vi "DOE Gas Volume Consumed.vi"() -> ()   [LabVIEW 2014]
uses:
  <vilib>/DAQmx/read.llb/DAQmx Read (Analog 1D DBL NChan 1Samp).vi
  <vilib>/DAQmx/miscellaneous.llb/DAQmx Fill In Error Info.vi
panel:
  out "25%Sum":dbl
  out "MaxRateSum":dbl
  out "25%RateTime":dbl
  out "MaxRateTime":dbl
  out "CurrentState":string
  in  "Data Sampling Rate (s)":dbl
  out "Second":dbl format="%#.0f"
  out "Minute":dbl format="%#.0f"
  out "25PercentInRange":bool
  out "25PercentRate":bool
  out "MaxRateState":bool
  out "25% Rate Run Average":dbl format="%#.3f"
  out "Target 25% Average":dbl format="%#.3f"
  out "Max Rate Run Avg.":dbl format="%#.3f"
  out "HV":dbl
  out "CF HR":dbl
  out "Meter SLPM":dbl
  out "Sum Time":dbl
  in  "Gas Type":string
  out "Current Meter":dbl
  in  "Reset":bool
  out "Seconds":dbl format="%#.0f"
  out "Minutes":dbl format="%#.0f"
  out "Cubic Ft. Flowed":dbl format="%#.3f"
  out "Signal 2":bool
  out "Reference6":dbl
  out "Reference5":dbl
  out "Reference4":dbl
  out "Reference3":dbl
  out "Reference2":dbl
  out "Reference1":dbl
  in  "HeatingValueLP":dbl=2450.0 min=2400.0 max=2600.0 step=1.0
  out "Output 6":dbl min=0.0 max=5.0 step=0.01
  out "Output 5":dbl min=0.0 max=5.0 step=0.01
  out "Output 4":dbl min=0.0 max=5.0 step=0.01
  out "Output 3":dbl min=0.0 max=5.0 step=0.01
  out "Output 2":dbl min=0.0 max=5.0 step=0.01
  out "Output 1":dbl min=0.0 max=5.0 step=0.01
  in  "HeatingValueNG":dbl=990.0 min=950.0 max=1050.0 step=1.0
  out "Flow Rate":dbl format="%#.0f"
  # "Instant Flow Rate (BTU/hr)"
  # "Heating Value"
  # "Signal"
  # "Elapsed Time"
  # ":"
  # "In Range"
  # "25% Rate Countdown Timer"
  # ":"
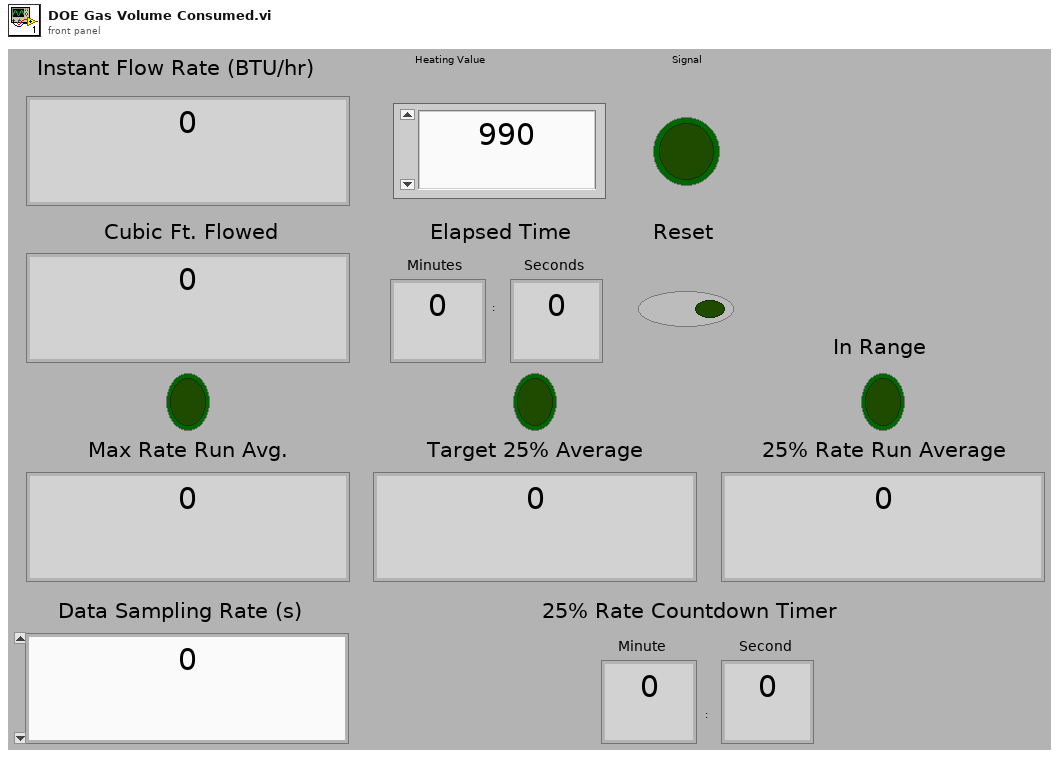
[diagram p1: front panel]
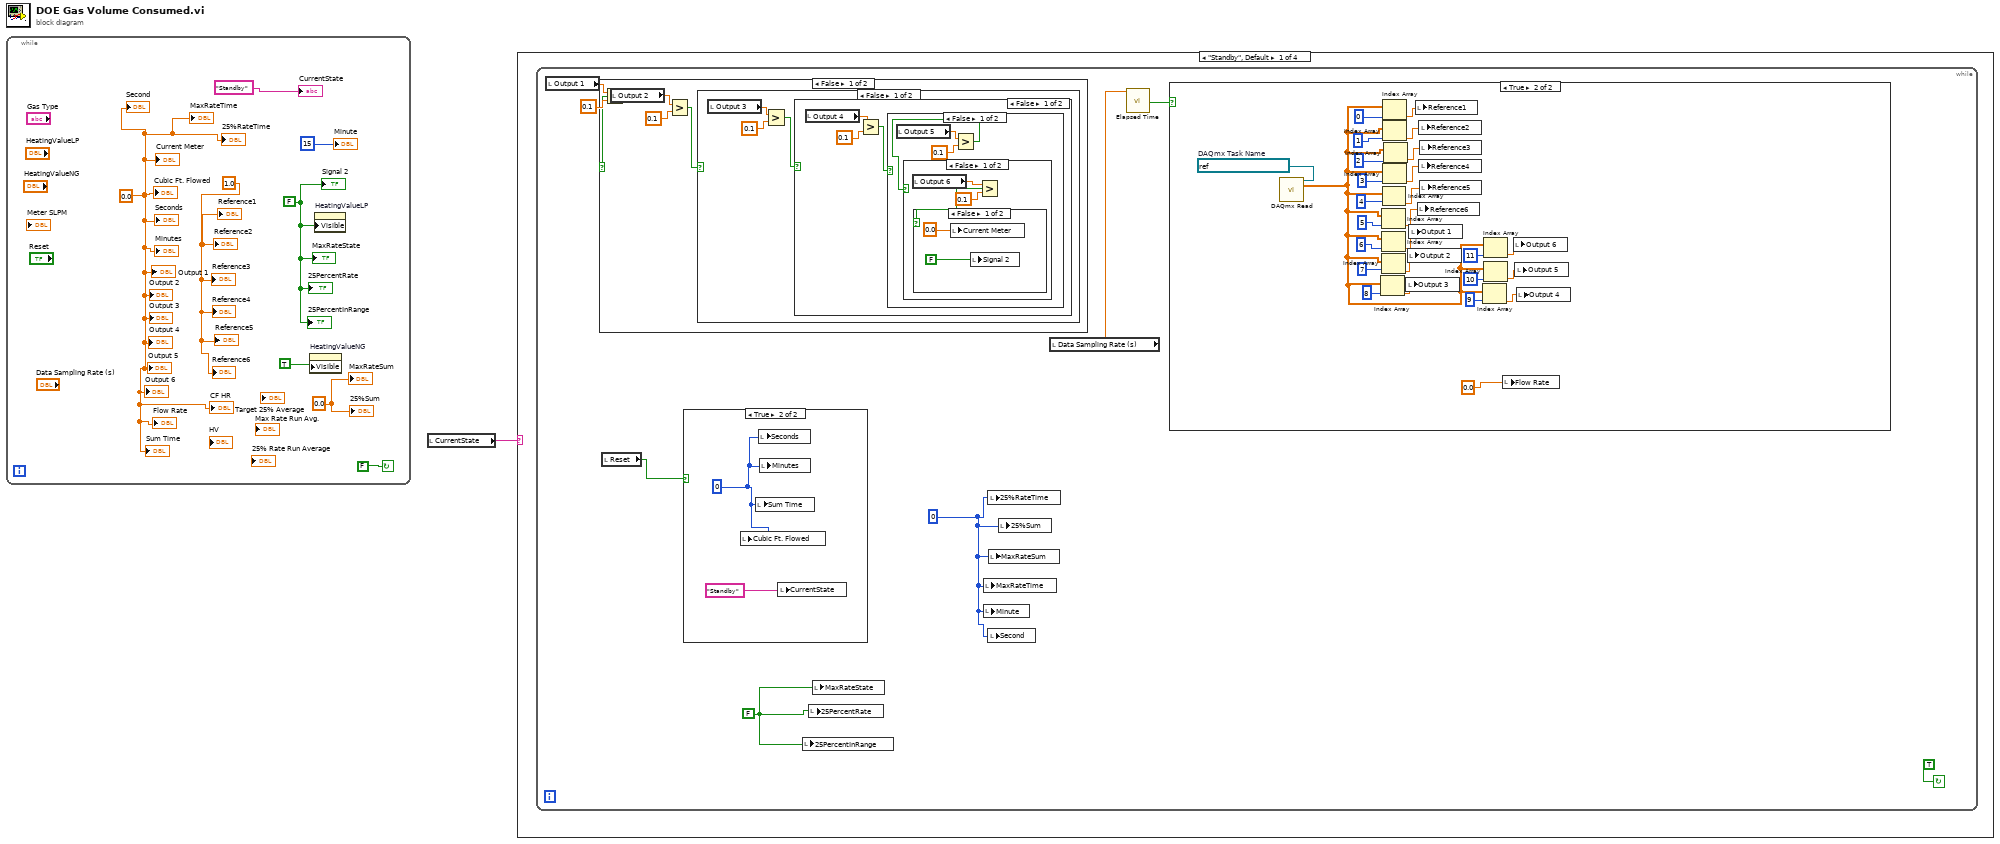
[diagram p0: block diagram]
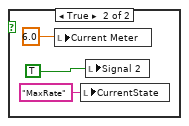
[diagram p3: hidden frame]
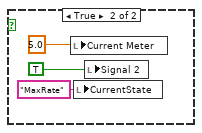
[diagram p4: hidden frame]
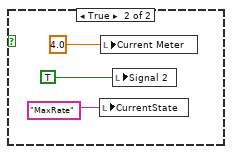
[diagram p5: hidden frame]
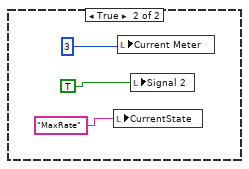
[diagram p6: hidden frame]
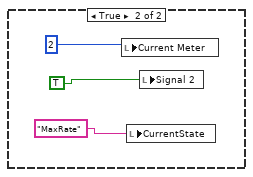
[diagram p7: hidden frame]
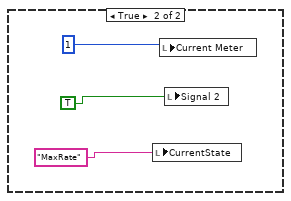
[diagram p8: hidden frame]
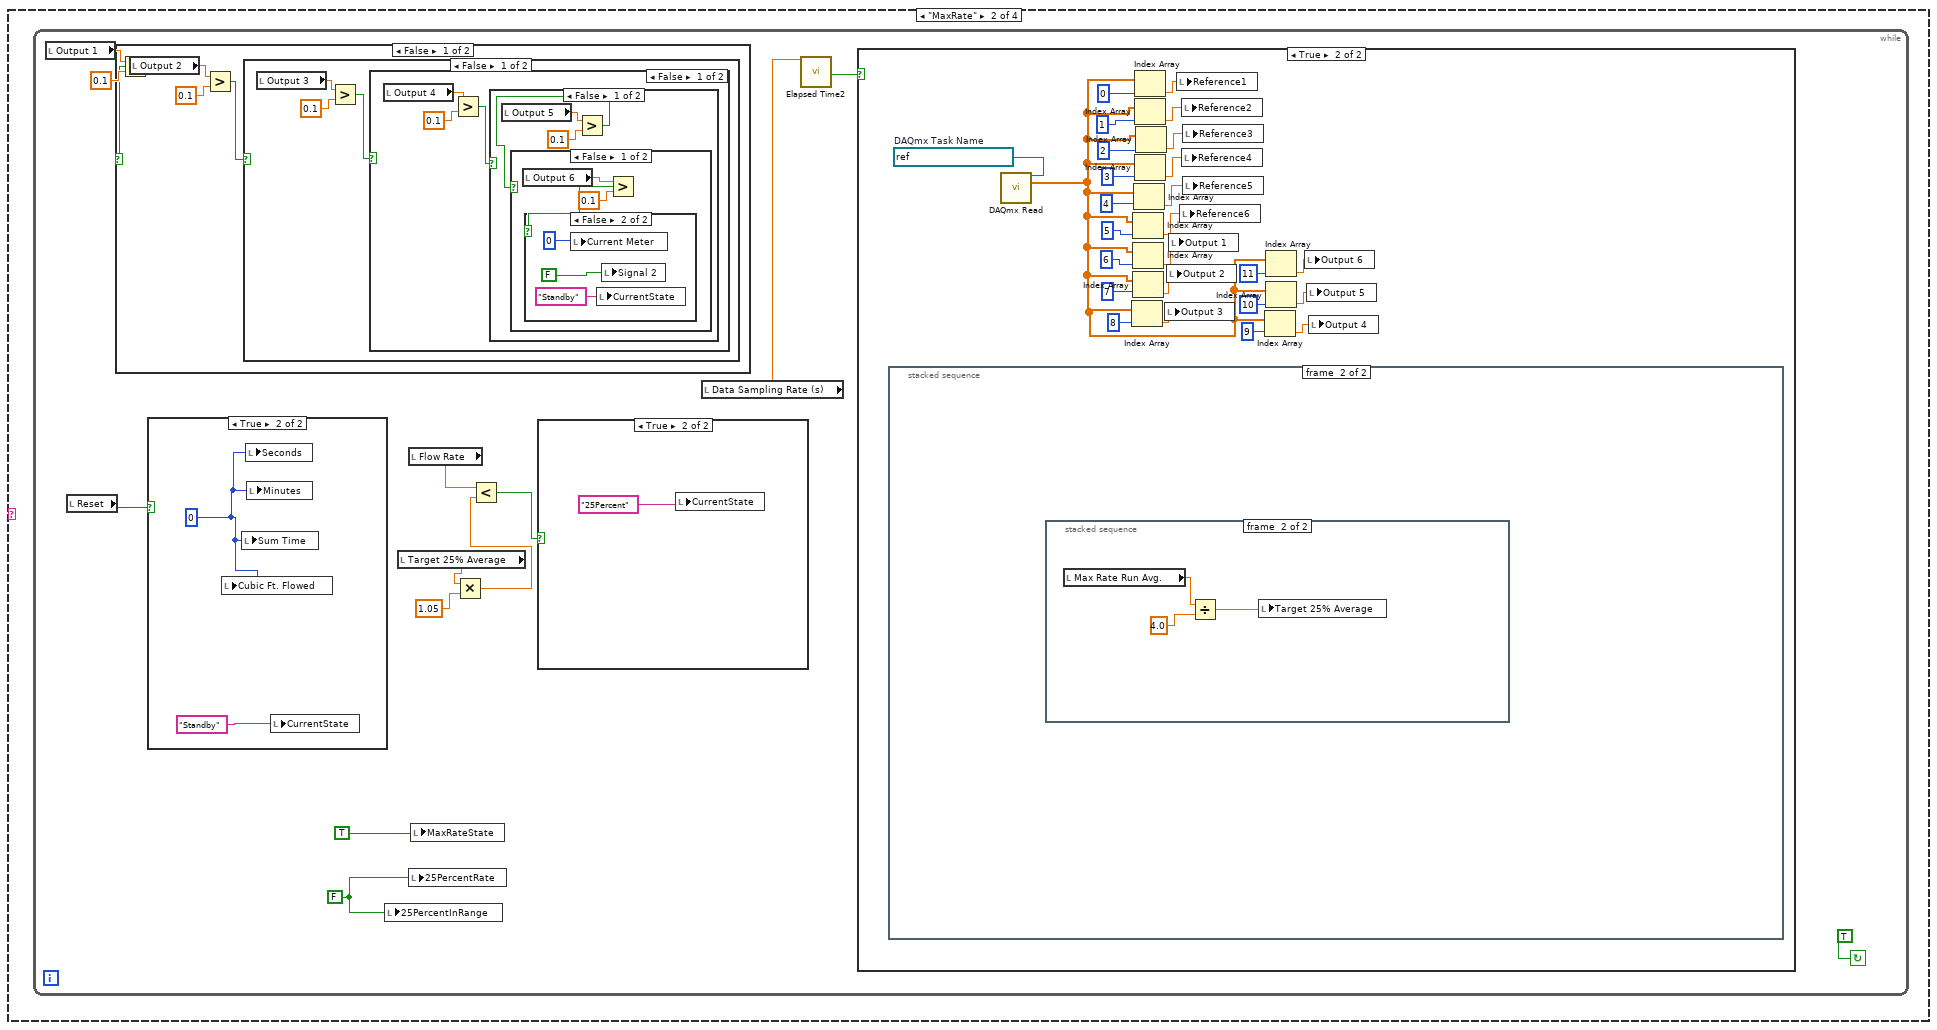
[diagram p10: hidden frame]
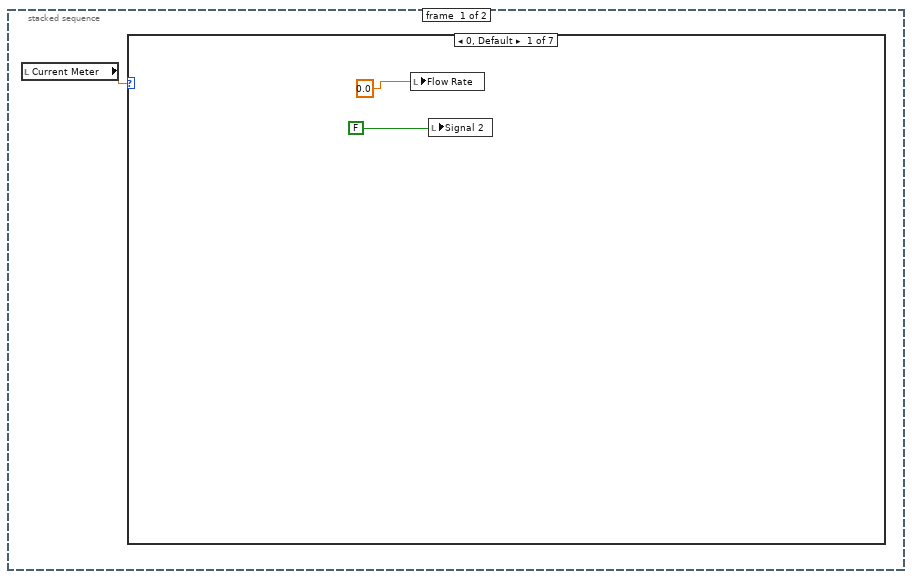
[diagram p13: hidden frame]
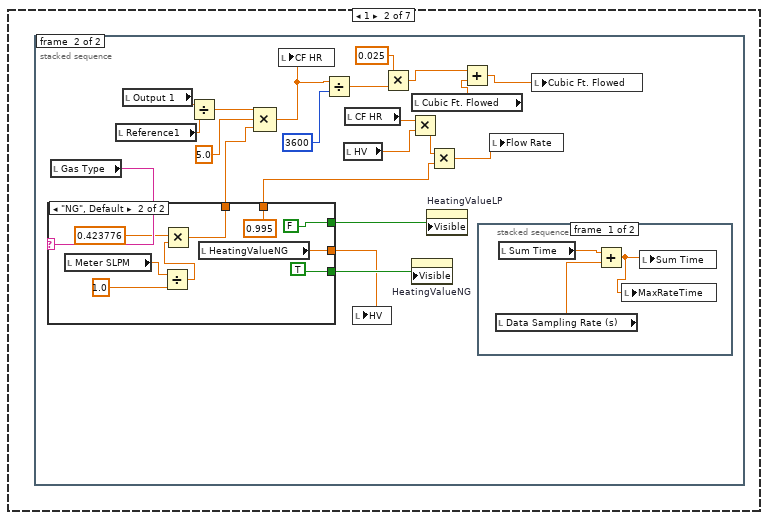
[diagram p14: hidden frame]
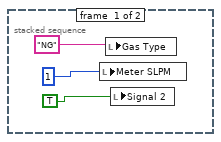
[diagram p15: hidden frame]
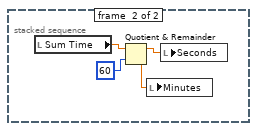
[diagram p16: hidden frame]
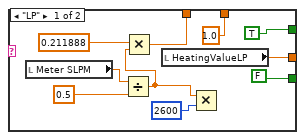
[diagram p17: hidden frame]
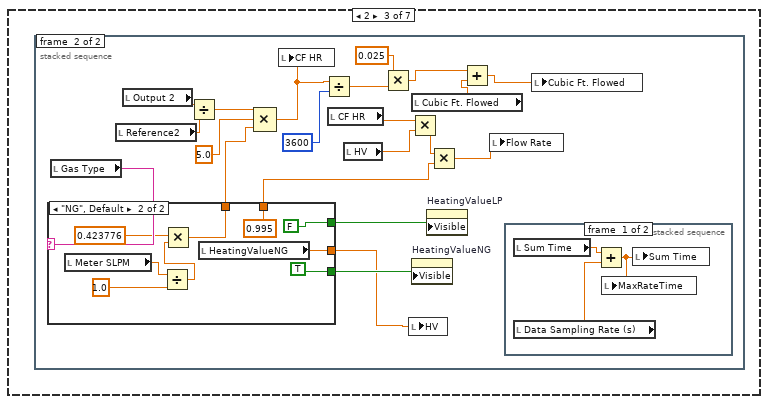
[diagram p18: hidden frame]
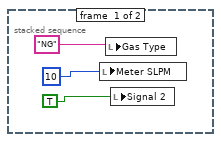
[diagram p19: hidden frame]
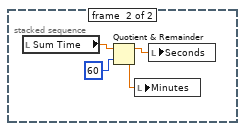
[diagram p20: hidden frame]
diagram:
  n1 = while {
    stop <- FALSE continue-if-true
    w2 = 0.0
    w6 = FALSE
    w9 = 1.0
    w3 = 0.0
    n2 = property on="HeatingValueNG" class="DigNum (strict)"("Visible"=TRUE) -> ()  [unwired: 2 in, 2 out]
    n3 = property on="HeatingValueLP" class="DigNum (strict)"("Visible"=w6) -> ()  [unwired: 2 in, 2 out]
    "Output 1" <- w3
    "Output 2" <- w3
    "Output 3" <- w3
    "Output 4" <- w3
    "Output 5" <- w3
    "Output 6" <- w3
    "Reference1" <- w9
    "Reference2" <- w9
    "Reference3" <- w9
    "Reference4" <- w9
    "Reference5" <- w9
    "Reference6" <- w9
    "Flow Rate" <- w3
    "Signal 2" <- w6
    "Cubic Ft. Flowed" <- w3
    "Minutes" <- w3
    "Seconds" <- w3
    "Current Meter" <- w3
    "Sum Time" <- w3
    "CF HR" <- w3
    "MaxRateState" <- w6
    "25PercentRate" <- w6
    "25PercentInRange" <- w6
    "Minute" <- 15
    "Second" <- w3
    "CurrentState" <- "Standby"
    "25%RateTime" <- w3
    "MaxRateTime" <- w3
    "25%Sum" <- w2
    "MaxRateSum" <- w2
  }
  n4 = local read "CurrentState"() -> (w1:string)
  n5 = case shown="\"Standby\", Default" w1 {
    frame "Standby", Default {
      n6 = while {
        stop <- TRUE continue-if-true
        w10 = 0
        w11 = FALSE
        n7 = local read "Output 1"() -> (w15:dbl)
        n8 = local read "Reset"() -> (w17:bool)
        n9 = Greater?(x=w15, y=0.1) -> (0:w14:bool)
        n10 = case shown="False" w14 {
          frame False {
            n11 = local read "Output 2"() -> (w47:dbl)
            n12 = Greater?(x=w47, y=0.1) -> (0:w46:bool)
            n13 = case shown="False" w46 {
              frame False {
                n14 = local read "Output 3"() -> (w50:dbl)
                n15 = Greater?(x=w50, y=0.1) -> (0:w49:bool)
                n16 = case shown="False" w49 {
                  frame False {
                    n17 = local read "Output 4"() -> (w54:dbl)
                    n18 = Greater?(x=w54, y=0.1) -> (0:w52:bool)
                    n19 = case shown="False" w52 {
                      frame False {
                        n20 = local read "Output 5"() -> (w57:dbl)
                        n21 = Greater?(x=w57, y=0.1) -> (0:w55:bool)
                        n22 = case shown="False" w55 {
                          frame False {
                            n23 = local read "Output 6"() -> (w59:dbl)
                            n24 = Greater?(x=w59, y=0.1) -> (0:w58:bool)
                            n25 = case shown="False" w58 {
                              frame False {
                                n26 = local write "Current Meter"(0.0) -> ()
                                n27 = local write "Signal 2"(FALSE) -> ()
                              }
                              frame True {
                                n28 = local write "Current Meter"(6.0) -> ()
                                n29 = local write "CurrentState"("MaxRate") -> ()
                                n30 = local write "Signal 2"(TRUE) -> ()
                              }
                            }
                          }
                          frame True {
                            n31 = local write "Current Meter"(5.0) -> ()
                            n32 = local write "CurrentState"("MaxRate") -> ()
                            n33 = local write "Signal 2"(TRUE) -> ()
                          }
                        }
                      }
                      frame True {
                        n34 = local write "CurrentState"("MaxRate") -> ()
                        n35 = local write "Current Meter"(4.0) -> ()
                        n36 = local write "Signal 2"(TRUE) -> ()
                      }
                    }
                  }
                  frame True {
                    n37 = local write "CurrentState"("MaxRate") -> ()
                    n38 = local write "Current Meter"(3) -> ()
                    n39 = local write "Signal 2"(TRUE) -> ()
                  }
                }
              }
              frame True {
                n40 = local write "Current Meter"(2) -> ()
                n41 = local write "CurrentState"("MaxRate") -> ()
                n42 = local write "Signal 2"(TRUE) -> ()
              }
            }
          }
          frame True {
            n43 = local write "CurrentState"("MaxRate") -> ()
            n44 = local write "Current Meter"(1) -> ()
            n45 = local write "Signal 2"(TRUE) -> ()
          }
        }
        n46 = case shown="True" w17 {
          frame False {
          }
          frame True {
            w82 = 0
            n47 = local write "Cubic Ft. Flowed"(w82) -> ()
            n48 = local write "Sum Time"(w82) -> ()
            n49 = local write "Seconds"(w82) -> ()
            n50 = local write "Minutes"(w82) -> ()
            n51 = local write "CurrentState"("Standby") -> ()
          }
        }
        n52 = local write "25PercentInRange"(w11) -> ()
        n53 = local write "25PercentRate"(w11) -> ()
        n54 = local write "MaxRateState"(w11) -> ()
        n55 = local write "MaxRateTime"(w10) -> ()
        n56 = local write "Minute"(w10) -> ()
        n57 = local write "25%RateTime"(w10) -> ()
        n58 = local write "Second"(w10) -> ()
        n59 = local write "MaxRateSum"(w10) -> ()
        n60 = local write "25%Sum"(w10) -> ()
        n61 = local read "Data Sampling Rate (s)"() -> (w12:dbl)
        n62 = call "Elapsed Time"("Time Target (s)"=w12) -> ("Time has Elapsed"=w13:bool)  [unwired: 11 in, 7 out]
        n63 = case shown="True" w13 {
          frame False {
          }
          frame True {
            w45 = refnum<k21> "ReadFlowMeterIn"  # DAQmx Task Name
            n64 = call-poly <vilib>:"DAQmx Read.vi"("task/channels in"=w45) -> ("data"=w44:dbl[])  [unwired: 12 in, 2 out]
            n65 = Index Array(array=w44, index=8) -> (element=w28:dbl)
            n66 = Index Array(array=w44, index=5) -> (element=w25:dbl)
            n67 = Index Array(array=w44, index=6) -> (element=w26:dbl)
            n68 = Index Array(array=w44, index=7) -> (element=w27:dbl)
            n69 = Index Array(array=w44, index=4) -> (element=w24:dbl)
            n70 = Index Array(array=w44, index=0) -> (element=w20:dbl)
            n71 = Index Array(array=w44, index=1) -> (element=w21:dbl)
            n72 = Index Array(array=w44, index=3) -> (element=w23:dbl)
            n73 = Index Array(array=w44, index=2) -> (element=w22:dbl)
            n74 = local write "Output 3"(w28) -> ()
            n75 = local write "Output 2"(w27) -> ()
            n76 = local write "Output 1"(w26) -> ()
            n77 = local write "Reference1"(w20) -> ()
            n78 = local write "Reference6"(w25) -> ()
            n79 = local write "Reference2"(w21) -> ()
            n80 = local write "Reference4"(w23) -> ()
            n81 = local write "Reference3"(w22) -> ()
            n82 = local write "Reference5"(w24) -> ()
            n83 = Index Array(array=w44, index=9) -> (element=w29:dbl)
            n84 = Index Array(array=w44, index=11) -> (element=w31:dbl)
            n85 = Index Array(array=w44, index=10) -> (element=w30:dbl)
            n86 = local write "Flow Rate"(0.0) -> ()
            n87 = local write "Output 6"(w31) -> ()
            n88 = local write "Output 5"(w30) -> ()
            n89 = local write "Output 4"(w29) -> ()
          }
        }
      }
    }
    frame "MaxRate" {
      n90 = while {
        stop <- TRUE continue-if-true
        w88 = FALSE
        n91 = local read "Output 1"() -> (w93:dbl)
        n92 = local read "Reset"() -> (w95:bool)
        n93 = Greater?(x=w93, y=0.1) -> (0:w92:bool)
        n94 = case shown="False" w92 {
          frame False {
            n95 = local read "Output 2"() -> (w436:dbl)
            n96 = Greater?(x=w436, y=0.1) -> (0:w435:bool)
            n97 = case shown="False" w435 {
              frame False {
                n98 = local read "Output 3"() -> (w439:dbl)
                n99 = Greater?(x=w439, y=0.1) -> (0:w438:bool)
                n100 = case shown="False" w438 {
                  frame False {
                    n101 = local read "Output 4"() -> (w443:dbl)
                    n102 = Greater?(x=w443, y=0.1) -> (0:w441:bool)
                    n103 = case shown="False" w441 {
                      frame False {
                        n104 = local read "Output 5"() -> (w446:dbl)
                        n105 = Greater?(x=w446, y=0.1) -> (0:w444:bool)
                        n106 = case shown="False" w444 {
                          frame False {
                            n107 = local read "Output 6"() -> (w448:dbl)
                            n108 = Greater?(x=w448, y=0.1) -> (0:w447:bool)
                            n109 = case shown="False" w447 {
                              frame True {
                                n110 = local write "Current Meter"(6.0) -> ()
                                n111 = local write "Signal 2"(TRUE) -> ()
                              }
                              frame False {
                                n112 = local write "Current Meter"(0) -> ()
                                n113 = local write "CurrentState"("Standby") -> ()
                                n114 = local write "Signal 2"(FALSE) -> ()
                              }
                            }
                          }
                          frame True {
                            n115 = local write "Current Meter"(5.0) -> ()
                            n116 = local write "Signal 2"(TRUE) -> ()
                          }
                        }
                      }
                      frame True {
                        n117 = local write "Current Meter"(4.0) -> ()
                        n118 = local write "Signal 2"(TRUE) -> ()
                      }
                    }
                  }
                  frame True {
                    n119 = local write "Current Meter"(3) -> ()
                    n120 = local write "Signal 2"(TRUE) -> ()
                  }
                }
              }
              frame True {
                n121 = local write "Current Meter"(2) -> ()
                n122 = local write "Signal 2"(TRUE) -> ()
              }
            }
          }
          frame True {
            n123 = local write "Current Meter"(1) -> ()
            n124 = local write "Signal 2"(TRUE) -> ()
          }
        }
        n125 = case shown="True" w95 {
          frame False {
          }
          frame True {
            w466 = 0
            n126 = local write "Cubic Ft. Flowed"(w466) -> ()
            n127 = local write "Sum Time"(w466) -> ()
            n128 = local write "Seconds"(w466) -> ()
            n129 = local write "Minutes"(w466) -> ()
            n130 = local write "CurrentState"("Standby") -> ()
          }
        }
        n131 = local write "25PercentInRange"(w88) -> ()
        n132 = local read "Target 25% Average"() -> (w85:dbl)
        n133 = local read "Flow Rate"() -> (w87:dbl)
        n134 = local write "25PercentRate"(w88) -> ()
        n135 = local write "MaxRateState"(TRUE) -> ()
        n136 = Multiply(x=w85, y=1.05) -> (x*y=w84:dbl)
        n137 = Less?(x=w87, y=w84) -> (x < y?=w83:bool)
        n138 = case shown="True" w83 {
          frame False {
          }
          frame True {
            n139 = local write "CurrentState"("25Percent") -> ()
          }
        }
        n140 = local read "Data Sampling Rate (s)"() -> (w90:dbl)
        n141 = call "Elapsed Time2"("Time Target (s)"=w90) -> ("Time has Elapsed"=w91:bool)  [unwired: 11 in, 7 out]
        n142 = case shown="True" w91 {
          frame False {
          }
          frame True {
            w123 = refnum<k21> "ReadFlowMeterIn"  # DAQmx Task Name
            n143 = stacked-sequence {
              frame #0 {
                n144 = local read "Current Meter"() -> (w124:dbl)
                n145 = case shown="0, Default" w124 {
                  frame 0, Default {
                    n146 = local write "Flow Rate"(0.0) -> ()
                    n147 = local write "Signal 2"(FALSE) -> ()
                  }
                  frame 1 {
                    n148 = stacked-sequence {
                      frame #0 {
                        n149 = local write "Meter SLPM"(1) -> ()
                        n150 = local write "Gas Type"("NG") -> ()
                        n151 = local write "Signal 2"(TRUE) -> ()
                      }
                      frame #1 {
                        n152 = local read "Gas Type"() -> (w142:string)
                        n153 = case shown="\"NG\", Default" w142 {
                          tunnel: [w164 w173] -> w141
                          tunnel: [TRUE FALSE] -> w140
                          tunnel: [FALSE TRUE] -> w139
                          tunnel: [1.0 0.995] -> w138
                          tunnel: [w158 w168] -> w137
                          frame "LP" {
                            n154 = local read "Meter SLPM"() -> (w166:dbl)
                            n155 = Divide(x=w166, y=0.5) -> (x/y=w159:dbl)
                            n156 = Multiply(x=0.211888, y=w159) -> (x*y=w164:dbl)
                            n157 = local read "HeatingValueLP"() -> (w158:dbl)
                            n158 = Multiply(x=w159, y=2600) -> ()  [unwired: 1 out]
                          }
                          frame "NG", Default {
                            n159 = local read "Meter SLPM"() -> (w175:dbl)
                            n160 = Divide(x=w175, y=1.0) -> (x/y=w169:dbl)
                            n161 = Multiply(x=0.423776, y=w169) -> (x*y=w173:dbl)
                            n162 = local read "HeatingValueNG"() -> (w168:dbl)
                          }
                        }
                        n163 = local read "Reference1"() -> (w145:dbl)
                        n164 = local read "Output 1"() -> (w146:dbl)
                        n165 = Divide(x=w146, y=w145) -> (x/y=w143:dbl)
                        n166 = Compound Arithmetic op=MULTIPLY(w143, 5.0, w141) -> (w136:dbl)
                        n167 = local write "CF HR"(w136) -> ()
                        n168 = Divide(x=w136, y=3600) -> (x/y=w134:dbl)
                        n169 = local read "HV"() -> (w148:dbl)
                        n170 = local read "CF HR"() -> (w147:dbl)
                        n171 = local write "HV"(w137) -> ()
                        n172 = Multiply(x=0.025, y=w134) -> (x*y=w131:dbl)
                        n173 = Multiply(x=w147, y=w148) -> (x*y=w149:dbl)
                        n174 = local read "Cubic Ft. Flowed"() -> (w132:dbl)
                        n175 = property on="HeatingValueNG" class="DigNum (strict)"("Visible"=w139) -> ()  [unwired: 2 in, 2 out]
                        n176 = property on="HeatingValueLP" class="DigNum (strict)"("Visible"=w140) -> ()  [unwired: 2 in, 2 out]
                        n177 = Multiply(x=w149, y=w138) -> (x*y=w150:dbl)
                        n178 = Add(x=w131, y=w132) -> (x+y=w130:dbl)
                        n179 = stacked-sequence {
                          frame #0 {
                            n180 = local read "Data Sampling Rate (s)"() -> (w152:dbl)
                            n181 = local read "Sum Time"() -> (w153:dbl)
                            n182 = Add(x=w153, y=w152) -> (x+y=w151:dbl)
                            n183 = local write "MaxRateTime"(w151) -> ()
                            n184 = local write "Sum Time"(w151) -> ()
                          }
                          frame #1 {
                            n185 = local read "Sum Time"() -> (w157:dbl)
                            n186 = Quotient & Remainder(x=w157, y=60) -> (x-y*floor(x/y)=w154:dbl, floor(x/y)=w155:dbl)
                            n187 = local write "Minutes"(w155) -> ()
                            n188 = local write "Seconds"(w154) -> ()
                          }
                        }
                        n189 = local write "Flow Rate"(w150) -> ()
                        n190 = local write "Cubic Ft. Flowed"(w130) -> ()
                      }
                    }
                  }
                  frame 2 {
                    n191 = stacked-sequence {
                      frame #0 {
                        n192 = local write "Meter SLPM"(10) -> ()
                        n193 = local write "Gas Type"("NG") -> ()
                        n194 = local write "Signal 2"(TRUE) -> ()
                      }
                      frame #1 {
                        n195 = local read "Gas Type"() -> (w192:string)
                        n196 = case shown="\"NG\", Default" w192 {
                          tunnel: [w214 w223] -> w191
                          tunnel: [TRUE FALSE] -> w190
                          tunnel: [FALSE TRUE] -> w189
                          tunnel: [1.0 0.995] -> w188
                          tunnel: [w208 w218] -> w187
                          frame "LP" {
                            n197 = local read "Meter SLPM"() -> (w216:dbl)
                            n198 = Divide(x=w216, y=0.5) -> (x/y=w209:dbl)
                            n199 = Multiply(x=0.211888, y=w209) -> (x*y=w214:dbl)
                            n200 = local read "HeatingValueLP"() -> (w208:dbl)
                            n201 = Multiply(x=w209, y=2600) -> ()  [unwired: 1 out]
                          }
                          frame "NG", Default {
                            n202 = local read "Meter SLPM"() -> (w225:dbl)
                            n203 = Divide(x=w225, y=1.0) -> (x/y=w219:dbl)
                            n204 = Multiply(x=0.423776, y=w219) -> (x*y=w223:dbl)
                            n205 = local read "HeatingValueNG"() -> (w218:dbl)
                          }
                        }
                        n206 = local read "Reference2"() -> (w195:dbl)
                        n207 = local read "Output 2"() -> (w196:dbl)
                        n208 = Divide(x=w196, y=w195) -> (x/y=w193:dbl)
                        n209 = Compound Arithmetic op=MULTIPLY(w193, 5.0, w191) -> (w186:dbl)
                        n210 = local write "CF HR"(w186) -> ()
                        n211 = Divide(x=w186, y=3600) -> (x/y=w184:dbl)
                        n212 = local read "CF HR"() -> (w197:dbl)
                        n213 = local read "HV"() -> (w198:dbl)
                        n214 = Multiply(x=0.025, y=w184) -> (x*y=w181:dbl)
                        n215 = local write "HV"(w187) -> ()
                        n216 = Multiply(x=w197, y=w198) -> (x*y=w199:dbl)
                        n217 = local read "Cubic Ft. Flowed"() -> (w182:dbl)
                        n218 = property on="HeatingValueNG" class="DigNum (strict)"("Visible"=w189) -> ()  [unwired: 2 in, 2 out]
                        n219 = property on="HeatingValueLP" class="DigNum (strict)"("Visible"=w190) -> ()  [unwired: 2 in, 2 out]
                        n220 = Multiply(x=w199, y=w188) -> (x*y=w200:dbl)
                        n221 = Add(x=w181, y=w182) -> (x+y=w180:dbl)
                        n222 = local write "Flow Rate"(w200) -> ()
                        n223 = stacked-sequence {
                          frame #0 {
                            n224 = local read "Sum Time"() -> (w203:dbl)
                            n225 = local read "Data Sampling Rate (s)"() -> (w202:dbl)
                            n226 = Add(x=w203, y=w202) -> (x+y=w201:dbl)
                            n227 = local write "MaxRateTime"(w201) -> ()
                            n228 = local write "Sum Time"(w201) -> ()
                          }
                          frame #1 {
                            n229 = local read "Sum Time"() -> (w207:dbl)
                            n230 = Quotient & Remainder(x=w207, y=60) -> (x-y*floor(x/y)=w204:dbl, floor(x/y)=w205:dbl)
                            n231 = local write "Minutes"(w205) -> ()
                            n232 = local write "Seconds"(w204) -> ()
                          }
                        }
                        n233 = local write "Cubic Ft. Flowed"(w180) -> ()
                      }
                    }
                  }
                  frame 3 {
                    n234 = stacked-sequence {
                      frame #0 {
                        n235 = local write "Meter SLPM"(20) -> ()
                        n236 = local write "Gas Type"("NG") -> ()
                        n237 = local write "Signal 2"(TRUE) -> ()
                      }
                      frame #1 {
                        n238 = local read "Gas Type"() -> (w242:string)
                        n239 = case shown="\"NG\", Default" w242 {
                          tunnel: [w264 w273] -> w241
                          tunnel: [TRUE FALSE] -> w240
                          tunnel: [FALSE TRUE] -> w239
                          tunnel: [1.0 0.995] -> w238
                          tunnel: [w258 w268] -> w237
                          frame "LP" {
                            n240 = local read "Meter SLPM"() -> (w266:dbl)
                            n241 = Divide(x=w266, y=0.5) -> (x/y=w259:dbl)
                            n242 = Multiply(x=0.211888, y=w259) -> (x*y=w264:dbl)
                            n243 = local read "HeatingValueLP"() -> (w258:dbl)
                            n244 = Multiply(x=w259, y=2600) -> ()  [unwired: 1 out]
                          }
                          frame "NG", Default {
                            n245 = local read "Meter SLPM"() -> (w275:dbl)
                            n246 = Divide(x=w275, y=1.0) -> (x/y=w269:dbl)
                            n247 = Multiply(x=0.423776, y=w269) -> (x*y=w273:dbl)
                            n248 = local read "HeatingValueNG"() -> (w268:dbl)
                          }
                        }
                        n249 = local read "Reference3"() -> (w245:dbl)
                        n250 = local read "Output 3"() -> (w246:dbl)
                        n251 = Divide(x=w246, y=w245) -> (x/y=w243:dbl)
                        n252 = Compound Arithmetic op=MULTIPLY(w243, 5.0, w241) -> (w236:dbl)
                        n253 = local write "CF HR"(w236) -> ()
                        n254 = Divide(x=w236, y=3600) -> (x/y=w234:dbl)
                        n255 = local read "CF HR"() -> (w247:dbl)
                        n256 = local read "HV"() -> (w248:dbl)
                        n257 = Multiply(x=0.025, y=w234) -> (x*y=w231:dbl)
                        n258 = local write "HV"(w237) -> ()
                        n259 = Multiply(x=w247, y=w248) -> (x*y=w249:dbl)
                        n260 = local read "Cubic Ft. Flowed"() -> (w232:dbl)
                        n261 = property on="HeatingValueNG" class="DigNum (strict)"("Visible"=w239) -> ()  [unwired: 2 in, 2 out]
                        n262 = property on="HeatingValueLP" class="DigNum (strict)"("Visible"=w240) -> ()  [unwired: 2 in, 2 out]
                        n263 = Multiply(x=w249, y=w238) -> (x*y=w250:dbl)
                        n264 = Add(x=w231, y=w232) -> (x+y=w230:dbl)
                        n265 = local write "Flow Rate"(w250) -> ()
                        n266 = stacked-sequence {
                          frame #0 {
                            n267 = local read "Data Sampling Rate (s)"() -> (w252:dbl)
                            n268 = local read "Sum Time"() -> (w253:dbl)
                            n269 = Add(x=w253, y=w252) -> (x+y=w251:dbl)
                            n270 = local write "MaxRateTime"(w251) -> ()
                            n271 = local write "Sum Time"(w251) -> ()
                          }
                          frame #1 {
                            n272 = local read "Sum Time"() -> (w257:dbl)
                            n273 = Quotient & Remainder(x=w257, y=60) -> (x-y*floor(x/y)=w254:dbl, floor(x/y)=w255:dbl)
                            n274 = local write "Minutes"(w255) -> ()
                            n275 = local write "Seconds"(w254) -> ()
                          }
                        }
                        n276 = local write "Cubic Ft. Flowed"(w230) -> ()
                      }
                    }
                  }
                  frame 4 {
                    n277 = stacked-sequence {
                      frame #0 {
                        n278 = local write "Meter SLPM"(50) -> ()
                        n279 = local write "Gas Type"("NG") -> ()
                        n280 = local write "Signal 2"(TRUE) -> ()
                      }
                      frame #1 {
                        n281 = local read "Gas Type"() -> (w292:string)
                        n282 = case shown="\"NG\", Default" w292 {
                          tunnel: [w314 w323] -> w291
                          tunnel: [TRUE FALSE] -> w290
                          tunnel: [FALSE TRUE] -> w289
                          tunnel: [1.0 0.995] -> w288
                          tunnel: [w308 w318] -> w287
                          frame "LP" {
                            n283 = local read "Meter SLPM"() -> (w316:dbl)
                            n284 = Divide(x=w316, y=0.5) -> (x/y=w309:dbl)
                            n285 = Multiply(x=0.211888, y=w309) -> (x*y=w314:dbl)
                            n286 = local read "HeatingValueLP"() -> (w308:dbl)
                            n287 = Multiply(x=w309, y=2600) -> ()  [unwired: 1 out]
                          }
                          frame "NG", Default {
                            n288 = local read "Meter SLPM"() -> (w325:dbl)
                            n289 = Divide(x=w325, y=1.0) -> (x/y=w319:dbl)
                            n290 = Multiply(x=0.423776, y=w319) -> (x*y=w323:dbl)
                            n291 = local read "HeatingValueNG"() -> (w318:dbl)
                          }
                        }
                        n292 = local read "Reference4"() -> (w295:dbl)
                        n293 = local read "Output 4"() -> (w296:dbl)
                        n294 = Divide(x=w296, y=w295) -> (x/y=w293:dbl)
                        n295 = Compound Arithmetic op=MULTIPLY(w293, 5.0, w291) -> (w286:dbl)
                        n296 = local write "CF HR"(w286) -> ()
                        n297 = Divide(x=w286, y=3600) -> (x/y=w284:dbl)
                        n298 = local read "CF HR"() -> (w297:dbl)
                        n299 = local read "HV"() -> (w298:dbl)
                        n300 = Multiply(x=0.025, y=w284) -> (x*y=w281:dbl)
                        n301 = local write "HV"(w287) -> ()
                        n302 = Multiply(x=w297, y=w298) -> (x*y=w299:dbl)
                        n303 = local read "Cubic Ft. Flowed"() -> (w282:dbl)
                        n304 = property on="HeatingValueNG" class="DigNum (strict)"("Visible"=w289) -> ()  [unwired: 2 in, 2 out]
                        n305 = property on="HeatingValueLP" class="DigNum (strict)"("Visible"=w290) -> ()  [unwired: 2 in, 2 out]
                        n306 = Multiply(x=w299, y=w288) -> (x*y=w300:dbl)
                        n307 = Add(x=w281, y=w282) -> (x+y=w280:dbl)
                        n308 = local write "Flow Rate"(w300) -> ()
                        n309 = stacked-sequence {
                          frame #0 {
                            n310 = local read "Sum Time"() -> (w303:dbl)
                            n311 = local read "Data Sampling Rate (s)"() -> (w302:dbl)
                            n312 = Add(x=w303, y=w302) -> (x+y=w301:dbl)
                            n313 = local write "MaxRateTime"(w301) -> ()
                            n314 = local write "Sum Time"(w301) -> ()
                          }
                          frame #1 {
                            n315 = local read "Sum Time"() -> (w307:dbl)
                            n316 = Quotient & Remainder(x=w307, y=60) -> (x-y*floor(x/y)=w304:dbl, floor(x/y)=w305:dbl)
                            n317 = local write "Minutes"(w305) -> ()
                            n318 = local write "Seconds"(w304) -> ()
                          }
                        }
                        n319 = local write "Cubic Ft. Flowed"(w280) -> ()
                      }
                    }
                  }
                  frame 5 {
                    n320 = stacked-sequence {
                      frame #0 {
                        n321 = local write "Meter SLPM"(10) -> ()
                        n322 = local write "Gas Type"("LP") -> ()
                        n323 = local write "Signal 2"(TRUE) -> ()
                      }
                      frame #1 {
                        n324 = local read "Gas Type"() -> (w342:string)
                        n325 = case shown="\"NG\", Default" w342 {
                          tunnel: [w364 w373] -> w341
                          tunnel: [TRUE FALSE] -> w340
                          tunnel: [FALSE TRUE] -> w339
                          tunnel: [1.0 0.995] -> w338
                          tunnel: [w358 w368] -> w337
                          frame "LP" {
                            n326 = local read "Meter SLPM"() -> (w366:dbl)
                            n327 = Divide(x=w366, y=0.5) -> (x/y=w359:dbl)
                            n328 = Multiply(x=0.211888, y=w359) -> (x*y=w364:dbl)
                            n329 = local read "HeatingValueLP"() -> (w358:dbl)
                            n330 = Multiply(x=w359, y=2600) -> ()  [unwired: 1 out]
                          }
                          frame "NG", Default {
                            n331 = local read "Meter SLPM"() -> (w375:dbl)
                            n332 = Divide(x=w375, y=1.0) -> (x/y=w369:dbl)
                            n333 = Multiply(x=0.423776, y=w369) -> (x*y=w373:dbl)
                            n334 = local read "HeatingValueNG"() -> (w368:dbl)
                          }
                        }
                        n335 = local read "Reference5"() -> (w345:dbl)
                        n336 = local read "Output 5"() -> (w346:dbl)
                        n337 = Divide(x=w346, y=w345) -> (x/y=w343:dbl)
                        n338 = Compound Arithmetic op=MULTIPLY(w343, 5.0, w341) -> (w336:dbl)
                        n339 = local write "CF HR"(w336) -> ()
                        n340 = Divide(x=w336, y=3600) -> (x/y=w334:dbl)
                        n341 = local read "CF HR"() -> (w347:dbl)
                        n342 = local read "HV"() -> (w348:dbl)
                        n343 = Multiply(x=0.025, y=w334) -> (x*y=w331:dbl)
                        n344 = local write "HV"(w337) -> ()
                        n345 = Multiply(x=w347, y=w348) -> (x*y=w349:dbl)
                        n346 = local read "Cubic Ft. Flowed"() -> (w332:dbl)
                        n347 = property on="HeatingValueNG" class="DigNum (strict)"("Visible"=w339) -> ()  [unwired: 2 in, 2 out]
                        n348 = property on="HeatingValueLP" class="DigNum (strict)"("Visible"=w340) -> ()  [unwired: 2 in, 2 out]
                        n349 = Multiply(x=w349, y=w338) -> (x*y=w350:dbl)
                        n350 = Add(x=w331, y=w332) -> (x+y=w330:dbl)
                        n351 = local write "Flow Rate"(w350) -> ()
                        n352 = stacked-sequence {
                          frame #0 {
                            n353 = local read "Sum Time"() -> (w353:dbl)
                            n354 = local read "Data Sampling Rate (s)"() -> (w352:dbl)
                            n355 = Add(x=w353, y=w352) -> (x+y=w351:dbl)
                            n356 = local write "MaxRateTime"(w351) -> ()
                            n357 = local write "Sum Time"(w351) -> ()
                          }
                          frame #1 {
                            n358 = local read "Sum Time"() -> (w357:dbl)
                            n359 = Quotient & Remainder(x=w357, y=60) -> (x-y*floor(x/y)=w354:dbl, floor(x/y)=w355:dbl)
                            n360 = local write "Minutes"(w355) -> ()
                            n361 = local write "Seconds"(w354) -> ()
                          }
                        }
                        n362 = local write "Cubic Ft. Flowed"(w330) -> ()
                      }
                    }
                  }
                  frame 6 {
                    n363 = stacked-sequence {
                      frame #0 {
                        n364 = local write "Meter SLPM"(20) -> ()
                        n365 = local write "Gas Type"("LP") -> ()
                        n366 = local write "Signal 2"(TRUE) -> ()
                      }
                      frame #1 {
                        n367 = local read "Gas Type"() -> (w392:string)
                        n368 = case shown="\"NG\", Default" w392 {
                          tunnel: [w414 w423] -> w391
                          tunnel: [TRUE FALSE] -> w390
                          tunnel: [FALSE TRUE] -> w389
                          tunnel: [1.0 0.995] -> w388
                          tunnel: [w408 w418] -> w387
                          frame "LP" {
                            n369 = local read "Meter SLPM"() -> (w416:dbl)
                            n370 = Divide(x=w416, y=0.5) -> (x/y=w409:dbl)
                            n371 = Multiply(x=0.211888, y=w409) -> (x*y=w414:dbl)
                            n372 = local read "HeatingValueLP"() -> (w408:dbl)
                            n373 = Multiply(x=w409, y=2600) -> ()  [unwired: 1 out]
                          }
                          frame "NG", Default {
                            n374 = local read "Meter SLPM"() -> (w425:dbl)
                            n375 = Divide(x=w425, y=1.0) -> (x/y=w419:dbl)
                            n376 = Multiply(x=0.423776, y=w419) -> (x*y=w423:dbl)
                            n377 = local read "HeatingValueNG"() -> (w418:dbl)
                          }
                        }
                        n378 = local read "Reference6"() -> (w395:dbl)
                        n379 = local read "Output 6"() -> (w396:dbl)
                        n380 = Divide(x=w396, y=w395) -> (x/y=w393:dbl)
                        n381 = Compound Arithmetic op=MULTIPLY(w393, 5.0, w391) -> (w386:dbl)
                        n382 = local write "CF HR"(w386) -> ()
                        n383 = Divide(x=w386, y=3600) -> (x/y=w384:dbl)
                        n384 = local read "CF HR"() -> (w397:dbl)
                        n385 = local read "HV"() -> (w398:dbl)
                        n386 = Multiply(x=0.025, y=w384) -> (x*y=w381:dbl)
                        n387 = local write "HV"(w387) -> ()
                        n388 = Multiply(x=w397, y=w398) -> (x*y=w399:dbl)
                        n389 = local read "Cubic Ft. Flowed"() -> (w382:dbl)
                        n390 = property on="HeatingValueNG" class="DigNum (strict)"("Visible"=w389) -> ()  [unwired: 2 in, 2 out]
                        n391 = property on="HeatingValueLP" class="DigNum (strict)"("Visible"=w390) -> ()  [unwired: 2 in, 2 out]
                        n392 = Multiply(x=w399, y=w388) -> (x*y=w400:dbl)
                        n393 = Add(x=w381, y=w382) -> (x+y=w380:dbl)
                        n394 = stacked-sequence {
                          frame #0 {
                            n395 = local read "Data Sampling Rate (s)"() -> (w402:dbl)
                            n396 = local read "Sum Time"() -> (w403:dbl)
                            n397 = Add(x=w403, y=w402) -> (x+y=w401:dbl)
                            n398 = local write "MaxRateTime"(w401) -> ()
                            n399 = local write "Sum Time"(w401) -> ()
                          }
                          frame #1 {
                            n400 = local read "Sum Time"() -> (w407:dbl)
                            n401 = Quotient & Remainder(x=w407, y=60) -> (x-y*floor(x/y)=w404:dbl, floor(x/y)=w405:dbl)
                            n402 = local write "Minutes"(w405) -> ()
                            n403 = local write "Seconds"(w404) -> ()
                          }
                        }
                        n404 = local write "Flow Rate"(w400) -> ()
                        n405 = local write "Cubic Ft. Flowed"(w380) -> ()
                      }
                    }
                  }
                }
              }
              frame #1 {
                n406 = stacked-sequence {
                  frame #0 {
                    n407 = local read "MaxRateSum"() -> (w430:dbl)
                    n408 = local read "Flow Rate"() -> (w431:dbl)
                    n409 = local read "MaxRateTime"() -> (w429:dbl)
                    n410 = Add(x=w431, y=w430) -> (x+y=w428:dbl)
                    n411 = Divide(x=w428, y=w429) -> (x/y=w427:dbl)
                    n412 = local write "Max Rate Run Avg."(w427) -> ()
                  }
                  frame #1 {
                    n413 = local read "Max Rate Run Avg."() -> (w434:dbl)
                    n414 = Divide(x=w434, y=4.0) -> (x/y=w432:dbl)
                    n415 = local write "Target 25% Average"(w432) -> ()
                  }
                }
              }
            }
            n416 = call-poly <vilib>:"DAQmx Read.vi"("task/channels in"=w123) -> ("data"=w122:dbl[])  [unwired: 12 in, 2 out]
            n417 = Index Array(array=w122, index=8) -> (element=w106:dbl)
            n418 = Index Array(array=w122, index=5) -> (element=w103:dbl)
            n419 = Index Array(array=w122, index=6) -> (element=w104:dbl)
            n420 = Index Array(array=w122, index=7) -> (element=w105:dbl)
            n421 = Index Array(array=w122, index=4) -> (element=w102:dbl)
            n422 = Index Array(array=w122, index=0) -> (element=w98:dbl)
            n423 = Index Array(array=w122, index=1) -> (element=w99:dbl)
            n424 = Index Array(array=w122, index=3) -> (element=w101:dbl)
            n425 = Index Array(array=w122, index=2) -> (element=w100:dbl)
            n426 = local write "Output 3"(w106) -> ()
            n427 = local write "Output 2"(w105) -> ()
            n428 = local write "Output 1"(w104) -> ()
            n429 = local write "Reference1"(w98) -> ()
            n430 = local write "Reference6"(w103) -> ()
            n431 = local write "Reference2"(w99) -> ()
            n432 = local write "Reference4"(w101) -> ()
            n433 = local write "Reference3"(w100) -> ()
            n434 = local write "Reference5"(w102) -> ()
            n435 = Index Array(array=w122, index=9) -> (element=w107:dbl)
            n436 = Index Array(array=w122, index=11) -> (element=w109:dbl)
            n437 = Index Array(array=w122, index=10) -> (element=w108:dbl)
            n438 = local write "Output 6"(w109) -> ()
            n439 = local write "Output 5"(w108) -> ()
            n440 = local write "Output 4"(w107) -> ()
          }
        }
      }
    }
    frame "25Percent" {
      n441 = while {
        stop <- TRUE continue-if-true
        n442 = local read "Output 1"() -> (w484:dbl)
        n443 = local read "Reset"() -> (w486:bool)
        n444 = Greater?(x=w484, y=0.1) -> (0:w483:bool)
        n445 = case shown="False" w483 {
          frame False {
            n446 = local read "Output 2"() -> (w829:dbl)
            n447 = Greater?(x=w829, y=0.1) -> (0:w828:bool)
            n448 = case shown="False" w828 {
              frame False {
                n449 = local read "Output 3"() -> (w832:dbl)
                n450 = Greater?(x=w832, y=0.1) -> (0:w831:bool)
                n451 = case shown="False" w831 {
                  frame False {
                    n452 = local read "Output 4"() -> (w836:dbl)
                    n453 = Greater?(x=w836, y=0.1) -> (0:w834:bool)
                    n454 = case shown="False" w834 {
                      frame False {
                        n455 = local read "Output 5"() -> (w839:dbl)
                        n456 = Greater?(x=w839, y=0.1) -> (0:w837:bool)
                        n457 = case shown="False" w837 {
                          frame False {
                            n458 = local read "Output 6"() -> (w841:dbl)
                            n459 = Greater?(x=w841, y=0.1) -> (0:w840:bool)
                            n460 = case shown="False" w840 {
                              frame True {
                                n461 = local write "Current Meter"(6.0) -> ()
                                n462 = local write "Signal 2"(TRUE) -> ()
                              }
                              frame False {
                                n463 = local write "Current Meter"(0) -> ()
                                n464 = local write "CurrentState"("Standby") -> ()
                                n465 = local write "Signal 2"(FALSE) -> ()
                              }
                            }
                          }
                          frame True {
                            n466 = local write "Current Meter"(5.0) -> ()
                            n467 = local write "Signal 2"(TRUE) -> ()
                          }
                        }
                      }
                      frame True {
                        n468 = local write "Current Meter"(4.0) -> ()
                        n469 = local write "Signal 2"(TRUE) -> ()
                      }
                    }
                  }
                  frame True {
                    n470 = local write "Current Meter"(3) -> ()
                    n471 = local write "Signal 2"(TRUE) -> ()
                  }
                }
              }
              frame True {
                n472 = local write "Current Meter"(2) -> ()
                n473 = local write "Signal 2"(TRUE) -> ()
              }
            }
          }
          frame True {
            n474 = local write "Current Meter"(1) -> ()
            n475 = local write "Signal 2"(TRUE) -> ()
          }
        }
        n476 = case shown="True" w486 {
          frame False {
          }
          frame True {
            w859 = 0
            n477 = local write "Cubic Ft. Flowed"(w859) -> ()
            n478 = local write "Sum Time"(w859) -> ()
            n479 = local write "Seconds"(w859) -> ()
            n480 = local write "Minutes"(w859) -> ()
            n481 = local write "CurrentState"("Standby") -> ()
          }
        }
        n482 = local read "Target 25% Average"() -> (w473:dbl)
        n483 = local read "Flow Rate"() -> (w476:dbl)
        n484 = local write "25PercentRate"(TRUE) -> ()
        n485 = local write "MaxRateState"(FALSE) -> ()
        n486 = local read "25%RateTime"() -> (w468:dbl)
        n487 = Multiply(x=w473, y=1.05) -> (x*y=w477:dbl)
        n488 = Less?(x=w476, y=w477) -> (x < y?=w471:bool)
        n489 = Greater Or Equal?(x=w468, y=900) -> (x >= y?=w467:bool)
        n490 = Multiply(x=w473, y=0.95) -> (x*y=w474:dbl)
        n491 = Greater?(x=w476, y=w474) -> (0:w472:bool)
        n492 = case shown="True" w467 {
          frame False {
          }
          frame True {
            n493 = local write "CurrentState"("Complete") -> ()
          }
        }
        n494 = And(x=w472, y=w471) -> (x .and. y?=w470:bool)
        n495 = local write "25PercentInRange"(w470) -> ()
        n496 = local read "Data Sampling Rate (s)"() -> (w481:dbl)
        n497 = call "Elapsed Time3"("Time Target (s)"=w481) -> ("Time has Elapsed"=w482:bool)  [unwired: 11 in, 7 out]
        n498 = case shown="True" w482 {
          frame False {
          }
          frame True {
            w514 = refnum<k21> "ReadFlowMeterIn"  # DAQmx Task Name
            n499 = stacked-sequence {
              frame #0 {
                n500 = local read "Current Meter"() -> (w515:dbl)
                n501 = case shown="6" w515 {
                  frame 0, Default {
                    n502 = local write "Flow Rate"(0.0) -> ()
                    n503 = local write "Signal 2"(FALSE) -> ()
                  }
                  frame 1 {
                    n504 = stacked-sequence {
                      frame #0 {
                        n505 = local write "Meter SLPM"(1) -> ()
                        n506 = local write "Gas Type"("NG") -> ()
                        n507 = local write "Signal 2"(TRUE) -> ()
                      }
                      frame #1 {
                        n508 = local read "Gas Type"() -> (w533:string)
                        n509 = case shown="\"NG\", Default" w533 {
                          tunnel: [w555 w564] -> w532
                          tunnel: [TRUE FALSE] -> w531
                          tunnel: [FALSE TRUE] -> w530
                          tunnel: [1.0 0.995] -> w529
                          tunnel: [w549 w559] -> w528
                          frame "LP" {
                            n510 = local read "Meter SLPM"() -> (w557:dbl)
                            n511 = Divide(x=w557, y=0.5) -> (x/y=w550:dbl)
                            n512 = Multiply(x=0.211888, y=w550) -> (x*y=w555:dbl)
                            n513 = local read "HeatingValueLP"() -> (w549:dbl)
                            n514 = Multiply(x=w550, y=2600) -> ()  [unwired: 1 out]
                          }
                          frame "NG", Default {
                            n515 = local read "Meter SLPM"() -> (w566:dbl)
                            n516 = Divide(x=w566, y=1.0) -> (x/y=w560:dbl)
                            n517 = Multiply(x=0.423776, y=w560) -> (x*y=w564:dbl)
                            n518 = local read "HeatingValueNG"() -> (w559:dbl)
                          }
                        }
                        n519 = local read "Reference1"() -> (w536:dbl)
                        n520 = local read "Output 1"() -> (w537:dbl)
                        n521 = Divide(x=w537, y=w536) -> (x/y=w534:dbl)
                        n522 = Compound Arithmetic op=MULTIPLY(w534, 5.0, w532) -> (w527:dbl)
                        n523 = local write "CF HR"(w527) -> ()
                        n524 = Divide(x=w527, y=3600) -> (x/y=w525:dbl)
                        n525 = local read "HV"() -> (w539:dbl)
                        n526 = local read "CF HR"() -> (w538:dbl)
                        n527 = local write "HV"(w528) -> ()
                        n528 = Multiply(x=0.025, y=w525) -> (x*y=w522:dbl)
                        n529 = Multiply(x=w538, y=w539) -> (x*y=w540:dbl)
                        n530 = local read "Cubic Ft. Flowed"() -> (w523:dbl)
                        n531 = property on="HeatingValueNG" class="DigNum (strict)"("Visible"=w530) -> ()  [unwired: 2 in, 2 out]
                        n532 = property on="HeatingValueLP" class="DigNum (strict)"("Visible"=w531) -> ()  [unwired: 2 in, 2 out]
                        n533 = Multiply(x=w540, y=w529) -> (x*y=w541:dbl)
                        n534 = Add(x=w522, y=w523) -> (x+y=w521:dbl)
                        n535 = stacked-sequence {
                          frame #0 {
                            n536 = local read "Data Sampling Rate (s)"() -> (w543:dbl)
                            n537 = local read "Sum Time"() -> (w544:dbl)
                            n538 = Add(x=w544, y=w543) -> (x+y=w542:dbl)
                            n539 = local write "25%RateTime"(w542) -> ()
                            n540 = local write "Sum Time"(w542) -> ()
                          }
                          frame #1 {
                            n541 = local read "Sum Time"() -> (w548:dbl)
                            n542 = Quotient & Remainder(x=w548, y=60) -> (x-y*floor(x/y)=w545:dbl, floor(x/y)=w546:dbl)
                            n543 = local write "Minutes"(w546) -> ()
                            n544 = local write "Seconds"(w545) -> ()
                          }
                        }
                        n545 = local write "Flow Rate"(w541) -> ()
                        n546 = local write "Cubic Ft. Flowed"(w521) -> ()
                      }
                    }
                  }
                  frame 2 {
                    n547 = stacked-sequence {
                      frame #0 {
                        n548 = local write "Meter SLPM"(10) -> ()
                        n549 = local write "Gas Type"("NG") -> ()
                        n550 = local write "Signal 2"(TRUE) -> ()
                      }
                      frame #1 {
                        n551 = local read "Gas Type"() -> (w583:string)
                        n552 = case shown="\"NG\", Default" w583 {
                          tunnel: [w605 w614] -> w582
                          tunnel: [TRUE FALSE] -> w581
                          tunnel: [FALSE TRUE] -> w580
                          tunnel: [1.0 0.995] -> w579
                          tunnel: [w599 w609] -> w578
                          frame "LP" {
                            n553 = local read "Meter SLPM"() -> (w607:dbl)
                            n554 = Divide(x=w607, y=0.5) -> (x/y=w600:dbl)
                            n555 = Multiply(x=0.211888, y=w600) -> (x*y=w605:dbl)
                            n556 = local read "HeatingValueLP"() -> (w599:dbl)
                            n557 = Multiply(x=w600, y=2600) -> ()  [unwired: 1 out]
                          }
                          frame "NG", Default {
                            n558 = local read "Meter SLPM"() -> (w616:dbl)
                            n559 = Divide(x=w616, y=1.0) -> (x/y=w610:dbl)
                            n560 = Multiply(x=0.423776, y=w610) -> (x*y=w614:dbl)
                            n561 = local read "HeatingValueNG"() -> (w609:dbl)
                          }
                        }
                        n562 = local read "Reference2"() -> (w586:dbl)
                        n563 = local read "Output 2"() -> (w587:dbl)
                        n564 = Divide(x=w587, y=w586) -> (x/y=w584:dbl)
                        n565 = Compound Arithmetic op=MULTIPLY(w584, 5.0, w582) -> (w577:dbl)
                        n566 = local write "CF HR"(w577) -> ()
                        n567 = Divide(x=w577, y=3600) -> (x/y=w575:dbl)
                        n568 = local read "CF HR"() -> (w588:dbl)
                        n569 = local read "HV"() -> (w589:dbl)
                        n570 = Multiply(x=0.025, y=w575) -> (x*y=w572:dbl)
                        n571 = local write "HV"(w578) -> ()
                        n572 = Multiply(x=w588, y=w589) -> (x*y=w590:dbl)
                        n573 = local read "Cubic Ft. Flowed"() -> (w573:dbl)
                        n574 = property on="HeatingValueNG" class="DigNum (strict)"("Visible"=w580) -> ()  [unwired: 2 in, 2 out]
                        n575 = property on="HeatingValueLP" class="DigNum (strict)"("Visible"=w581) -> ()  [unwired: 2 in, 2 out]
                        n576 = Multiply(x=w590, y=w579) -> (x*y=w591:dbl)
                        n577 = Add(x=w572, y=w573) -> (x+y=w571:dbl)
                        n578 = local write "Flow Rate"(w591) -> ()
                        n579 = stacked-sequence {
                          frame #0 {
                            n580 = local read "Sum Time"() -> (w594:dbl)
                            n581 = local read "Data Sampling Rate (s)"() -> (w593:dbl)
                            n582 = Add(x=w594, y=w593) -> (x+y=w592:dbl)
                            n583 = local write "25%RateTime"(w592) -> ()
                            n584 = local write "Sum Time"(w592) -> ()
                          }
                          frame #1 {
                            n585 = local read "Sum Time"() -> (w598:dbl)
                            n586 = Quotient & Remainder(x=w598, y=60) -> (x-y*floor(x/y)=w595:dbl, floor(x/y)=w596:dbl)
                            n587 = local write "Minutes"(w596) -> ()
                            n588 = local write "Seconds"(w595) -> ()
                          }
                        }
                        n589 = local write "Cubic Ft. Flowed"(w571) -> ()
                      }
                    }
                  }
                  frame 3 {
                    n590 = stacked-sequence {
                      frame #0 {
                        n591 = local write "Meter SLPM"(20) -> ()
                        n592 = local write "Gas Type"("NG") -> ()
                        n593 = local write "Signal 2"(TRUE) -> ()
                      }
                      frame #1 {
                        n594 = local read "Gas Type"() -> (w633:string)
                        n595 = case shown="\"NG\", Default" w633 {
                          tunnel: [w655 w664] -> w632
                          tunnel: [TRUE FALSE] -> w631
                          tunnel: [FALSE TRUE] -> w630
                          tunnel: [1.0 0.995] -> w629
                          tunnel: [w649 w659] -> w628
                          frame "LP" {
                            n596 = local read "Meter SLPM"() -> (w657:dbl)
                            n597 = Divide(x=w657, y=0.5) -> (x/y=w650:dbl)
                            n598 = Multiply(x=0.211888, y=w650) -> (x*y=w655:dbl)
                            n599 = local read "HeatingValueLP"() -> (w649:dbl)
                            n600 = Multiply(x=w650, y=2600) -> ()  [unwired: 1 out]
                          }
                          frame "NG", Default {
                            n601 = local read "Meter SLPM"() -> (w666:dbl)
                            n602 = Divide(x=w666, y=1.0) -> (x/y=w660:dbl)
                            n603 = Multiply(x=0.423776, y=w660) -> (x*y=w664:dbl)
                            n604 = local read "HeatingValueNG"() -> (w659:dbl)
                          }
                        }
                        n605 = local read "Reference3"() -> (w636:dbl)
                        n606 = local read "Output 3"() -> (w637:dbl)
                        n607 = Divide(x=w637, y=w636) -> (x/y=w634:dbl)
                        n608 = Compound Arithmetic op=MULTIPLY(w634, 5.0, w632) -> (w627:dbl)
                        n609 = local write "CF HR"(w627) -> ()
                        n610 = Divide(x=w627, y=3600) -> (x/y=w625:dbl)
                        n611 = local read "CF HR"() -> (w638:dbl)
                        n612 = local read "HV"() -> (w639:dbl)
                        n613 = Multiply(x=0.025, y=w625) -> (x*y=w622:dbl)
                        n614 = local write "HV"(w628) -> ()
                        n615 = Multiply(x=w638, y=w639) -> (x*y=w640:dbl)
                        n616 = local read "Cubic Ft. Flowed"() -> (w623:dbl)
                        n617 = property on="HeatingValueNG" class="DigNum (strict)"("Visible"=w630) -> ()  [unwired: 2 in, 2 out]
                        n618 = property on="HeatingValueLP" class="DigNum (strict)"("Visible"=w631) -> ()  [unwired: 2 in, 2 out]
                        n619 = Multiply(x=w640, y=w629) -> (x*y=w641:dbl)
                        n620 = Add(x=w622, y=w623) -> (x+y=w621:dbl)
                        n621 = local write "Flow Rate"(w641) -> ()
                        n622 = stacked-sequence {
                          frame #0 {
                            n623 = local read "Data Sampling Rate (s)"() -> (w643:dbl)
                            n624 = local read "Sum Time"() -> (w644:dbl)
                            n625 = Add(x=w644, y=w643) -> (x+y=w642:dbl)
                            n626 = local write "25%RateTime"(w642) -> ()
                            n627 = local write "Sum Time"(w642) -> ()
                          }
                          frame #1 {
                            n628 = local read "Sum Time"() -> (w648:dbl)
                            n629 = Quotient & Remainder(x=w648, y=60) -> (x-y*floor(x/y)=w645:dbl, floor(x/y)=w646:dbl)
                            n630 = local write "Minutes"(w646) -> ()
                            n631 = local write "Seconds"(w645) -> ()
                          }
                        }
                        n632 = local write "Cubic Ft. Flowed"(w621) -> ()
                      }
                    }
                  }
                  frame 4 {
                    n633 = stacked-sequence {
                      frame #0 {
                        n634 = local write "Meter SLPM"(50) -> ()
                        n635 = local write "Gas Type"("NG") -> ()
                        n636 = local write "Signal 2"(TRUE) -> ()
                      }
                      frame #1 {
                        n637 = local read "Gas Type"() -> (w683:string)
                        n638 = case shown="\"NG\", Default" w683 {
                          tunnel: [w705 w714] -> w682
                          tunnel: [TRUE FALSE] -> w681
                          tunnel: [FALSE TRUE] -> w680
                          tunnel: [1.0 0.995] -> w679
                          tunnel: [w699 w709] -> w678
                          frame "LP" {
                            n639 = local read "Meter SLPM"() -> (w707:dbl)
                            n640 = Divide(x=w707, y=0.5) -> (x/y=w700:dbl)
                            n641 = Multiply(x=0.211888, y=w700) -> (x*y=w705:dbl)
                            n642 = local read "HeatingValueLP"() -> (w699:dbl)
                            n643 = Multiply(x=w700, y=2600) -> ()  [unwired: 1 out]
                          }
                          frame "NG", Default {
                            n644 = local read "Meter SLPM"() -> (w716:dbl)
                            n645 = Divide(x=w716, y=1.0) -> (x/y=w710:dbl)
                            n646 = Multiply(x=0.423776, y=w710) -> (x*y=w714:dbl)
                            n647 = local read "HeatingValueNG"() -> (w709:dbl)
                          }
                        }
                        n648 = local read "Reference4"() -> (w686:dbl)
                        n649 = local read "Output 4"() -> (w687:dbl)
                        n650 = Divide(x=w687, y=w686) -> (x/y=w684:dbl)
                        n651 = Compound Arithmetic op=MULTIPLY(w684, 5.0, w682) -> (w677:dbl)
                        n652 = local write "CF HR"(w677) -> ()
                        n653 = Divide(x=w677, y=3600) -> (x/y=w675:dbl)
                        n654 = local read "CF HR"() -> (w688:dbl)
                        n655 = local read "HV"() -> (w689:dbl)
                        n656 = Multiply(x=0.025, y=w675) -> (x*y=w672:dbl)
                        n657 = local write "HV"(w678) -> ()
                        n658 = Multiply(x=w688, y=w689) -> (x*y=w690:dbl)
                        n659 = local read "Cubic Ft. Flowed"() -> (w673:dbl)
                        n660 = property on="HeatingValueNG" class="DigNum (strict)"("Visible"=w680) -> ()  [unwired: 2 in, 2 out]
                        n661 = property on="HeatingValueLP" class="DigNum (strict)"("Visible"=w681) -> ()  [unwired: 2 in, 2 out]
                        n662 = Multiply(x=w690, y=w679) -> (x*y=w691:dbl)
                        n663 = Add(x=w672, y=w673) -> (x+y=w671:dbl)
                        n664 = local write "Flow Rate"(w691) -> ()
                        n665 = stacked-sequence {
                          frame #0 {
                            n666 = local read "Sum Time"() -> (w694:dbl)
                            n667 = local read "Data Sampling Rate (s)"() -> (w693:dbl)
                            n668 = Add(x=w694, y=w693) -> (x+y=w692:dbl)
                            n669 = local write "25%RateTime"(w692) -> ()
                            n670 = local write "Sum Time"(w692) -> ()
                          }
                          frame #1 {
                            n671 = local read "Sum Time"() -> (w698:dbl)
                            n672 = Quotient & Remainder(x=w698, y=60) -> (x-y*floor(x/y)=w695:dbl, floor(x/y)=w696:dbl)
                            n673 = local write "Minutes"(w696) -> ()
                            n674 = local write "Seconds"(w695) -> ()
                          }
                        }
                        n675 = local write "Cubic Ft. Flowed"(w671) -> ()
                      }
                    }
                  }
                  frame 5 {
                    n676 = stacked-sequence {
                      frame #0 {
                        n677 = local write "Meter SLPM"(10) -> ()
                        n678 = local write "Gas Type"("LP") -> ()
                        n679 = local write "Signal 2"(TRUE) -> ()
                      }
                      frame #1 {
                        n680 = local read "Gas Type"() -> (w733:string)
                        n681 = case shown="\"NG\", Default" w733 {
                          tunnel: [w755 w764] -> w732
                          tunnel: [TRUE FALSE] -> w731
                          tunnel: [FALSE TRUE] -> w730
                          tunnel: [1.0 0.995] -> w729
                          tunnel: [w749 w759] -> w728
                          frame "LP" {
                            n682 = local read "Meter SLPM"() -> (w757:dbl)
                            n683 = Divide(x=w757, y=0.5) -> (x/y=w750:dbl)
                            n684 = Multiply(x=0.211888, y=w750) -> (x*y=w755:dbl)
                            n685 = local read "HeatingValueLP"() -> (w749:dbl)
                            n686 = Multiply(x=w750, y=2600) -> ()  [unwired: 1 out]
                          }
                          frame "NG", Default {
                            n687 = local read "Meter SLPM"() -> (w766:dbl)
                            n688 = Divide(x=w766, y=1.0) -> (x/y=w760:dbl)
                            n689 = Multiply(x=0.423776, y=w760) -> (x*y=w764:dbl)
                            n690 = local read "HeatingValueNG"() -> (w759:dbl)
                          }
                        }
                        n691 = local read "Reference5"() -> (w736:dbl)
                        n692 = local read "Output 5"() -> (w737:dbl)
                        n693 = Divide(x=w737, y=w736) -> (x/y=w734:dbl)
                        n694 = Compound Arithmetic op=MULTIPLY(w734, 5.0, w732) -> (w727:dbl)
                        n695 = local write "CF HR"(w727) -> ()
                        n696 = Divide(x=w727, y=3600) -> (x/y=w725:dbl)
                        n697 = local read "CF HR"() -> (w738:dbl)
                        n698 = local read "HV"() -> (w739:dbl)
                        n699 = Multiply(x=0.025, y=w725) -> (x*y=w722:dbl)
                        n700 = local write "HV"(w728) -> ()
                        n701 = Multiply(x=w738, y=w739) -> (x*y=w740:dbl)
                        n702 = local read "Cubic Ft. Flowed"() -> (w723:dbl)
                        n703 = property on="HeatingValueNG" class="DigNum (strict)"("Visible"=w730) -> ()  [unwired: 2 in, 2 out]
                        n704 = property on="HeatingValueLP" class="DigNum (strict)"("Visible"=w731) -> ()  [unwired: 2 in, 2 out]
                        n705 = Multiply(x=w740, y=w729) -> (x*y=w741:dbl)
                        n706 = Add(x=w722, y=w723) -> (x+y=w721:dbl)
                        n707 = local write "Flow Rate"(w741) -> ()
                        n708 = stacked-sequence {
                          frame #0 {
                            n709 = local read "Sum Time"() -> (w744:dbl)
                            n710 = local read "Data Sampling Rate (s)"() -> (w743:dbl)
                            n711 = Add(x=w744, y=w743) -> (x+y=w742:dbl)
                            n712 = local write "25%RateTime"(w742) -> ()
                            n713 = local write "Sum Time"(w742) -> ()
                          }
                          frame #1 {
                            n714 = local read "Sum Time"() -> (w748:dbl)
                            n715 = Quotient & Remainder(x=w748, y=60) -> (x-y*floor(x/y)=w745:dbl, floor(x/y)=w746:dbl)
                            n716 = local write "Minutes"(w746) -> ()
                            n717 = local write "Seconds"(w745) -> ()
                          }
                        }
                        n718 = local write "Cubic Ft. Flowed"(w721) -> ()
                      }
                    }
                  }
                  frame 6 {
                    n719 = stacked-sequence {
                      frame #0 {
                        n720 = local write "Meter SLPM"(20) -> ()
                        n721 = local write "Gas Type"("LP") -> ()
                        n722 = local write "Signal 2"(TRUE) -> ()
                      }
                      frame #1 {
                        n723 = local read "Gas Type"() -> (w783:string)
                        n724 = case shown="\"NG\", Default" w783 {
                          tunnel: [w805 w814] -> w782
                          tunnel: [TRUE FALSE] -> w781
                          tunnel: [FALSE TRUE] -> w780
                          tunnel: [1.0 0.995] -> w779
                          tunnel: [w799 w809] -> w778
                          frame "LP" {
                            n725 = local read "Meter SLPM"() -> (w807:dbl)
                            n726 = Divide(x=w807, y=0.5) -> (x/y=w800:dbl)
                            n727 = Multiply(x=0.211888, y=w800) -> (x*y=w805:dbl)
                            n728 = local read "HeatingValueLP"() -> (w799:dbl)
                            n729 = Multiply(x=w800, y=2600) -> ()  [unwired: 1 out]
                          }
                          frame "NG", Default {
                            n730 = local read "Meter SLPM"() -> (w816:dbl)
                            n731 = Divide(x=w816, y=1.0) -> (x/y=w810:dbl)
                            n732 = Multiply(x=0.423776, y=w810) -> (x*y=w814:dbl)
                            n733 = local read "HeatingValueNG"() -> (w809:dbl)
                          }
                        }
                        n734 = local read "Reference6"() -> (w786:dbl)
                        n735 = local read "Output 6"() -> (w787:dbl)
                        n736 = Divide(x=w787, y=w786) -> (x/y=w784:dbl)
                        n737 = Compound Arithmetic op=MULTIPLY(w784, 5.0, w782) -> (w777:dbl)
                        n738 = local write "CF HR"(w777) -> ()
                        n739 = Divide(x=w777, y=3600) -> (x/y=w775:dbl)
                        n740 = local read "CF HR"() -> (w788:dbl)
                        n741 = local read "HV"() -> (w789:dbl)
                        n742 = Multiply(x=0.025, y=w775) -> (x*y=w772:dbl)
                        n743 = local write "HV"(w778) -> ()
                        n744 = Multiply(x=w788, y=w789) -> (x*y=w790:dbl)
                        n745 = local read "Cubic Ft. Flowed"() -> (w773:dbl)
                        n746 = property on="HeatingValueNG" class="DigNum (strict)"("Visible"=w780) -> ()  [unwired: 2 in, 2 out]
                        n747 = property on="HeatingValueLP" class="DigNum (strict)"("Visible"=w781) -> ()  [unwired: 2 in, 2 out]
                        n748 = Multiply(x=w790, y=w779) -> (x*y=w791:dbl)
                        n749 = Add(x=w772, y=w773) -> (x+y=w771:dbl)
                        n750 = stacked-sequence {
                          frame #0 {
                            n751 = local read "Data Sampling Rate (s)"() -> (w793:dbl)
                            n752 = local read "Sum Time"() -> (w794:dbl)
                            n753 = Add(x=w794, y=w793) -> (x+y=w792:dbl)
                            n754 = local write "25%RateTime"(w792) -> ()
                            n755 = local write "Sum Time"(w792) -> ()
                          }
                          frame #1 {
                            n756 = local read "Sum Time"() -> (w798:dbl)
                            n757 = Quotient & Remainder(x=w798, y=60) -> (x-y*floor(x/y)=w795:dbl, floor(x/y)=w796:dbl)
                            n758 = local write "Minutes"(w796) -> ()
                            n759 = local write "Seconds"(w795) -> ()
                          }
                        }
                        n760 = local write "Flow Rate"(w791) -> ()
                        n761 = local write "Cubic Ft. Flowed"(w771) -> ()
                      }
                    }
                  }
                }
              }
              frame #1 {
                n762 = local read "25%Sum"() -> (w826:dbl)
                n763 = local read "Flow Rate"() -> (w827:dbl)
                n764 = local read "25%RateTime"() -> (w823:dbl)
                n765 = Add(x=w827, y=w826) -> (x+y=w825:dbl)
                n766 = Divide(x=w825, y=w823) -> (x/y=w824:dbl)
                n767 = Subtract(x=900.0, y=w823) -> (x-y=w820:dbl)
                n768 = Quotient & Remainder(x=w820, y=60) -> (x-y*floor(x/y)=w818:dbl, floor(x/y)=w819:dbl)
                n769 = local write "Minute"(w819) -> ()
                n770 = local write "25% Rate Run Average"(w824) -> ()
                n771 = local write "Second"(w818) -> ()
              }
            }
            n772 = call-poly <vilib>:"DAQmx Read.vi"("task/channels in"=w514) -> ("data"=w513:dbl[])  [unwired: 12 in, 2 out]
            n773 = Index Array(array=w513, index=8) -> (element=w497:dbl)
            n774 = Index Array(array=w513, index=5) -> (element=w494:dbl)
            n775 = Index Array(array=w513, index=6) -> (element=w495:dbl)
            n776 = Index Array(array=w513, index=7) -> (element=w496:dbl)
            n777 = Index Array(array=w513, index=4) -> (element=w493:dbl)
            n778 = Index Array(array=w513, index=0) -> (element=w489:dbl)
            n779 = Index Array(array=w513, index=1) -> (element=w490:dbl)
            n780 = Index Array(array=w513, index=3) -> (element=w492:dbl)
            n781 = Index Array(array=w513, index=2) -> (element=w491:dbl)
            n782 = local write "Output 3"(w497) -> ()
            n783 = local write "Output 2"(w496) -> ()
            n784 = local write "Output 1"(w495) -> ()
            n785 = local write "Reference1"(w489) -> ()
            n786 = local write "Reference6"(w494) -> ()
            n787 = local write "Reference2"(w490) -> ()
            n788 = local write "Reference4"(w492) -> ()
            n789 = local write "Reference3"(w491) -> ()
            n790 = local write "Reference5"(w493) -> ()
            n791 = Index Array(array=w513, index=9) -> (element=w498:dbl)
            n792 = Index Array(array=w513, index=11) -> (element=w500:dbl)
            n793 = Index Array(array=w513, index=10) -> (element=w499:dbl)
            n794 = local write "Output 6"(w500) -> ()
            n795 = local write "Output 5"(w499) -> ()
            n796 = local write "Output 4"(w498) -> ()
          }
        }
      }
    }
    frame "Complete" {
      n797 = while {
        stop <- TRUE continue-if-true
        w860 = FALSE
        n798 = local read "Output 1"() -> (w864:dbl)
        n799 = local read "Reset"() -> (w866:bool)
        n800 = Greater?(x=w864, y=0.1) -> (0:w863:bool)
        n801 = case shown="False" w863 {
          frame False {
            n802 = local read "Output 2"() -> (w1198:dbl)
            n803 = Greater?(x=w1198, y=0.1) -> (0:w1197:bool)
            n804 = case shown="False" w1197 {
              frame False {
                n805 = local read "Output 3"() -> (w1201:dbl)
                n806 = Greater?(x=w1201, y=0.1) -> (0:w1200:bool)
                n807 = case shown="False" w1200 {
                  frame False {
                    n808 = local read "Output 4"() -> (w1205:dbl)
                    n809 = Greater?(x=w1205, y=0.1) -> (0:w1203:bool)
                    n810 = case shown="False" w1203 {
                      frame False {
                        n811 = local read "Output 5"() -> (w1208:dbl)
                        n812 = Greater?(x=w1208, y=0.1) -> (0:w1206:bool)
                        n813 = case shown="False" w1206 {
                          frame False {
                            n814 = local read "Output 6"() -> (w1210:dbl)
                            n815 = Greater?(x=w1210, y=0.1) -> (0:w1209:bool)
                            n816 = case shown="False" w1209 {
                              frame True {
                                n817 = local write "Current Meter"(6.0) -> ()
                                n818 = local write "Signal 2"(TRUE) -> ()
                              }
                              frame False {
                                n819 = local write "Current Meter"(0) -> ()
                                n820 = local write "CurrentState"("Standby") -> ()
                                n821 = local write "Signal 2"(FALSE) -> ()
                              }
                            }
                          }
                          frame True {
                            n822 = local write "Current Meter"(5.0) -> ()
                            n823 = local write "Signal 2"(TRUE) -> ()
                          }
                        }
                      }
                      frame True {
                        n824 = local write "Current Meter"(4.0) -> ()
                        n825 = local write "Signal 2"(TRUE) -> ()
                      }
                    }
                  }
                  frame True {
                    n826 = local write "Current Meter"(3) -> ()
                    n827 = local write "Signal 2"(TRUE) -> ()
                  }
                }
              }
              frame True {
                n828 = local write "Current Meter"(2) -> ()
                n829 = local write "Signal 2"(TRUE) -> ()
              }
            }
          }
          frame True {
            n830 = local write "Current Meter"(1) -> ()
            n831 = local write "Signal 2"(TRUE) -> ()
          }
        }
        n832 = case shown="True" w866 {
          frame False {
          }
          frame True {
            w1228 = 0
            n833 = local write "Cubic Ft. Flowed"(w1228) -> ()
            n834 = local write "Sum Time"(w1228) -> ()
            n835 = local write "Seconds"(w1228) -> ()
            n836 = local write "Minutes"(w1228) -> ()
            n837 = local write "CurrentState"("Standby") -> ()
          }
        }
        n838 = local write "25PercentInRange"(w860) -> ()
        n839 = local write "25PercentRate"(w860) -> ()
        n840 = local write "MaxRateState"(w860) -> ()
        n841 = local read "Data Sampling Rate (s)"() -> (w861:dbl)
        n842 = call "Elapsed Time4"("Time Target (s)"=w861) -> ("Time has Elapsed"=w862:bool)  [unwired: 11 in, 7 out]
        n843 = case shown="True" w862 {
          frame False {
          }
          frame True {
            w893 = refnum<k21> "ReadFlowMeterIn"  # DAQmx Task Name
            n844 = stacked-sequence {
              frame #0 {
                n845 = local read "Current Meter"() -> (w894:dbl)
                n846 = case shown="1" w894 {
                  frame 0, Default {
                    n847 = local write "Flow Rate"(0.0) -> ()
                    n848 = local write "Signal 2"(FALSE) -> ()
                  }
                  frame 1 {
                    n849 = stacked-sequence {
                      frame #0 {
                        n850 = local write "Meter SLPM"(1) -> ()
                        n851 = local write "Gas Type"("NG") -> ()
                        n852 = local write "Signal 2"(TRUE) -> ()
                      }
                      frame #1 {
                        n853 = local read "Gas Type"() -> (w912:string)
                        n854 = case shown="\"NG\", Default" w912 {
                          tunnel: [w934 w943] -> w911
                          tunnel: [TRUE FALSE] -> w910
                          tunnel: [FALSE TRUE] -> w909
                          tunnel: [1.0 0.995] -> w908
                          tunnel: [w928 w938] -> w907
                          frame "LP" {
                            n855 = local read "Meter SLPM"() -> (w936:dbl)
                            n856 = Divide(x=w936, y=0.5) -> (x/y=w929:dbl)
                            n857 = Multiply(x=0.211888, y=w929) -> (x*y=w934:dbl)
                            n858 = local read "HeatingValueLP"() -> (w928:dbl)
                            n859 = Multiply(x=w929, y=2600) -> ()  [unwired: 1 out]
                          }
                          frame "NG", Default {
                            n860 = local read "Meter SLPM"() -> (w945:dbl)
                            n861 = Divide(x=w945, y=1.0) -> (x/y=w939:dbl)
                            n862 = Multiply(x=0.423776, y=w939) -> (x*y=w943:dbl)
                            n863 = local read "HeatingValueNG"() -> (w938:dbl)
                          }
                        }
                        n864 = local read "Reference1"() -> (w915:dbl)
                        n865 = local read "Output 1"() -> (w916:dbl)
                        n866 = Divide(x=w916, y=w915) -> (x/y=w913:dbl)
                        n867 = Compound Arithmetic op=MULTIPLY(w913, 5.0, w911) -> (w906:dbl)
                        n868 = local write "CF HR"(w906) -> ()
                        n869 = Divide(x=w906, y=3600) -> (x/y=w904:dbl)
                        n870 = local read "HV"() -> (w918:dbl)
                        n871 = local read "CF HR"() -> (w917:dbl)
                        n872 = local write "HV"(w907) -> ()
                        n873 = Multiply(x=0.025, y=w904) -> (x*y=w901:dbl)
                        n874 = Multiply(x=w917, y=w918) -> (x*y=w919:dbl)
                        n875 = local read "Cubic Ft. Flowed"() -> (w902:dbl)
                        n876 = property on="HeatingValueNG" class="DigNum (strict)"("Visible"=w909) -> ()  [unwired: 2 in, 2 out]
                        n877 = property on="HeatingValueLP" class="DigNum (strict)"("Visible"=w910) -> ()  [unwired: 2 in, 2 out]
                        n878 = Multiply(x=w919, y=w908) -> (x*y=w920:dbl)
                        n879 = Add(x=w901, y=w902) -> (x+y=w900:dbl)
                        n880 = stacked-sequence {
                          frame #0 {
                            n881 = local read "Data Sampling Rate (s)"() -> (w922:dbl)
                            n882 = local read "Sum Time"() -> (w923:dbl)
                            n883 = Add(x=w923, y=w922) -> (x+y=w921:dbl)
                            n884 = local write "25%RateTime"(w921) -> ()
                            n885 = local write "Sum Time"(w921) -> ()
                          }
                          frame #1 {
                            n886 = local read "Sum Time"() -> (w927:dbl)
                            n887 = Quotient & Remainder(x=w927, y=60) -> (x-y*floor(x/y)=w924:dbl, floor(x/y)=w925:dbl)
                            n888 = local write "Minutes"(w925) -> ()
                            n889 = local write "Seconds"(w924) -> ()
                          }
                        }
                        n890 = local write "Flow Rate"(w920) -> ()
                        n891 = local write "Cubic Ft. Flowed"(w900) -> ()
                      }
                    }
                  }
                  frame 2 {
                    n892 = stacked-sequence {
                      frame #0 {
                        n893 = local write "Meter SLPM"(10) -> ()
                        n894 = local write "Gas Type"("NG") -> ()
                        n895 = local write "Signal 2"(TRUE) -> ()
                      }
                      frame #1 {
                        n896 = local read "Gas Type"() -> (w962:string)
                        n897 = case shown="\"NG\", Default" w962 {
                          tunnel: [w984 w993] -> w961
                          tunnel: [TRUE FALSE] -> w960
                          tunnel: [FALSE TRUE] -> w959
                          tunnel: [1.0 0.995] -> w958
                          tunnel: [w978 w988] -> w957
                          frame "LP" {
                            n898 = local read "Meter SLPM"() -> (w986:dbl)
                            n899 = Divide(x=w986, y=0.5) -> (x/y=w979:dbl)
                            n900 = Multiply(x=0.211888, y=w979) -> (x*y=w984:dbl)
                            n901 = local read "HeatingValueLP"() -> (w978:dbl)
                            n902 = Multiply(x=w979, y=2600) -> ()  [unwired: 1 out]
                          }
                          frame "NG", Default {
                            n903 = local read "Meter SLPM"() -> (w995:dbl)
                            n904 = Divide(x=w995, y=1.0) -> (x/y=w989:dbl)
                            n905 = Multiply(x=0.423776, y=w989) -> (x*y=w993:dbl)
                            n906 = local read "HeatingValueNG"() -> (w988:dbl)
                          }
                        }
                        n907 = local read "Reference2"() -> (w965:dbl)
                        n908 = local read "Output 2"() -> (w966:dbl)
                        n909 = Divide(x=w966, y=w965) -> (x/y=w963:dbl)
                        n910 = Compound Arithmetic op=MULTIPLY(w963, 5.0, w961) -> (w956:dbl)
                        n911 = local write "CF HR"(w956) -> ()
                        n912 = Divide(x=w956, y=3600) -> (x/y=w954:dbl)
                        n913 = local read "CF HR"() -> (w967:dbl)
                        n914 = local read "HV"() -> (w968:dbl)
                        n915 = Multiply(x=0.025, y=w954) -> (x*y=w951:dbl)
                        n916 = local write "HV"(w957) -> ()
                        n917 = Multiply(x=w967, y=w968) -> (x*y=w969:dbl)
                        n918 = local read "Cubic Ft. Flowed"() -> (w952:dbl)
                        n919 = property on="HeatingValueNG" class="DigNum (strict)"("Visible"=w959) -> ()  [unwired: 2 in, 2 out]
                        n920 = property on="HeatingValueLP" class="DigNum (strict)"("Visible"=w960) -> ()  [unwired: 2 in, 2 out]
                        n921 = Multiply(x=w969, y=w958) -> (x*y=w970:dbl)
                        n922 = Add(x=w951, y=w952) -> (x+y=w950:dbl)
                        n923 = local write "Flow Rate"(w970) -> ()
                        n924 = stacked-sequence {
                          frame #0 {
                            n925 = local read "Sum Time"() -> (w973:dbl)
                            n926 = local read "Data Sampling Rate (s)"() -> (w972:dbl)
                            n927 = Add(x=w973, y=w972) -> (x+y=w971:dbl)
                            n928 = local write "25%RateTime"(w971) -> ()
                            n929 = local write "Sum Time"(w971) -> ()
                          }
                          frame #1 {
                            n930 = local read "Sum Time"() -> (w977:dbl)
                            n931 = Quotient & Remainder(x=w977, y=60) -> (x-y*floor(x/y)=w974:dbl, floor(x/y)=w975:dbl)
                            n932 = local write "Minutes"(w975) -> ()
                            n933 = local write "Seconds"(w974) -> ()
                          }
                        }
                        n934 = local write "Cubic Ft. Flowed"(w950) -> ()
                      }
                    }
                  }
                  frame 3 {
                    n935 = stacked-sequence {
                      frame #0 {
                        n936 = local write "Meter SLPM"(20) -> ()
                        n937 = local write "Gas Type"("NG") -> ()
                        n938 = local write "Signal 2"(TRUE) -> ()
                      }
                      frame #1 {
                        n939 = local read "Gas Type"() -> (w1012:string)
                        n940 = case shown="\"NG\", Default" w1012 {
                          tunnel: [w1034 w1043] -> w1011
                          tunnel: [TRUE FALSE] -> w1010
                          tunnel: [FALSE TRUE] -> w1009
                          tunnel: [1.0 0.995] -> w1008
                          tunnel: [w1028 w1038] -> w1007
                          frame "LP" {
                            n941 = local read "Meter SLPM"() -> (w1036:dbl)
                            n942 = Divide(x=w1036, y=0.5) -> (x/y=w1029:dbl)
                            n943 = Multiply(x=0.211888, y=w1029) -> (x*y=w1034:dbl)
                            n944 = local read "HeatingValueLP"() -> (w1028:dbl)
                            n945 = Multiply(x=w1029, y=2600) -> ()  [unwired: 1 out]
                          }
                          frame "NG", Default {
                            n946 = local read "Meter SLPM"() -> (w1045:dbl)
                            n947 = Divide(x=w1045, y=1.0) -> (x/y=w1039:dbl)
                            n948 = Multiply(x=0.423776, y=w1039) -> (x*y=w1043:dbl)
                            n949 = local read "HeatingValueNG"() -> (w1038:dbl)
                          }
                        }
                        n950 = local read "Reference3"() -> (w1015:dbl)
                        n951 = local read "Output 3"() -> (w1016:dbl)
                        n952 = Divide(x=w1016, y=w1015) -> (x/y=w1013:dbl)
                        n953 = Compound Arithmetic op=MULTIPLY(w1013, 5.0, w1011) -> (w1006:dbl)
                        n954 = local write "CF HR"(w1006) -> ()
                        n955 = Divide(x=w1006, y=3600) -> (x/y=w1004:dbl)
                        n956 = local read "CF HR"() -> (w1017:dbl)
                        n957 = local read "HV"() -> (w1018:dbl)
                        n958 = Multiply(x=0.025, y=w1004) -> (x*y=w1001:dbl)
                        n959 = local write "HV"(w1007) -> ()
                        n960 = Multiply(x=w1017, y=w1018) -> (x*y=w1019:dbl)
                        n961 = local read "Cubic Ft. Flowed"() -> (w1002:dbl)
                        n962 = property on="HeatingValueNG" class="DigNum (strict)"("Visible"=w1009) -> ()  [unwired: 2 in, 2 out]
                        n963 = property on="HeatingValueLP" class="DigNum (strict)"("Visible"=w1010) -> ()  [unwired: 2 in, 2 out]
                        n964 = Multiply(x=w1019, y=w1008) -> (x*y=w1020:dbl)
                        n965 = Add(x=w1001, y=w1002) -> (x+y=w1000:dbl)
                        n966 = local write "Flow Rate"(w1020) -> ()
                        n967 = stacked-sequence {
                          frame #0 {
                            n968 = local read "Data Sampling Rate (s)"() -> (w1022:dbl)
                            n969 = local read "Sum Time"() -> (w1023:dbl)
                            n970 = Add(x=w1023, y=w1022) -> (x+y=w1021:dbl)
                            n971 = local write "25%RateTime"(w1021) -> ()
                            n972 = local write "Sum Time"(w1021) -> ()
                          }
                          frame #1 {
                            n973 = local read "Sum Time"() -> (w1027:dbl)
                            n974 = Quotient & Remainder(x=w1027, y=60) -> (x-y*floor(x/y)=w1024:dbl, floor(x/y)=w1025:dbl)
                            n975 = local write "Minutes"(w1025) -> ()
                            n976 = local write "Seconds"(w1024) -> ()
                          }
                        }
                        n977 = local write "Cubic Ft. Flowed"(w1000) -> ()
                      }
                    }
                  }
                  frame 4 {
                    n978 = stacked-sequence {
                      frame #0 {
                        n979 = local write "Meter SLPM"(50) -> ()
                        n980 = local write "Gas Type"("NG") -> ()
                        n981 = local write "Signal 2"(TRUE) -> ()
                      }
                      frame #1 {
                        n982 = local read "Gas Type"() -> (w1062:string)
                        n983 = case shown="\"NG\", Default" w1062 {
                          tunnel: [w1084 w1093] -> w1061
                          tunnel: [TRUE FALSE] -> w1060
                          tunnel: [FALSE TRUE] -> w1059
                          tunnel: [1.0 0.995] -> w1058
                          tunnel: [w1078 w1088] -> w1057
                          frame "LP" {
                            n984 = local read "Meter SLPM"() -> (w1086:dbl)
                            n985 = Divide(x=w1086, y=0.5) -> (x/y=w1079:dbl)
                            n986 = Multiply(x=0.211888, y=w1079) -> (x*y=w1084:dbl)
                            n987 = local read "HeatingValueLP"() -> (w1078:dbl)
                            n988 = Multiply(x=w1079, y=2600) -> ()  [unwired: 1 out]
                          }
                          frame "NG", Default {
                            n989 = local read "Meter SLPM"() -> (w1095:dbl)
                            n990 = Divide(x=w1095, y=1.0) -> (x/y=w1089:dbl)
                            n991 = Multiply(x=0.423776, y=w1089) -> (x*y=w1093:dbl)
                            n992 = local read "HeatingValueNG"() -> (w1088:dbl)
                          }
                        }
                        n993 = local read "Reference4"() -> (w1065:dbl)
                        n994 = local read "Output 4"() -> (w1066:dbl)
                        n995 = Divide(x=w1066, y=w1065) -> (x/y=w1063:dbl)
                        n996 = Compound Arithmetic op=MULTIPLY(w1063, 5.0, w1061) -> (w1056:dbl)
                        n997 = local write "CF HR"(w1056) -> ()
                        n998 = Divide(x=w1056, y=3600) -> (x/y=w1054:dbl)
                        n999 = local read "CF HR"() -> (w1067:dbl)
                        n1000 = local read "HV"() -> (w1068:dbl)
                        n1001 = Multiply(x=0.025, y=w1054) -> (x*y=w1051:dbl)
                        n1002 = local write "HV"(w1057) -> ()
                        n1003 = Multiply(x=w1067, y=w1068) -> (x*y=w1069:dbl)
                        n1004 = local read "Cubic Ft. Flowed"() -> (w1052:dbl)
                        n1005 = property on="HeatingValueNG" class="DigNum (strict)"("Visible"=w1059) -> ()  [unwired: 2 in, 2 out]
                        n1006 = property on="HeatingValueLP" class="DigNum (strict)"("Visible"=w1060) -> ()  [unwired: 2 in, 2 out]
                        n1007 = Multiply(x=w1069, y=w1058) -> (x*y=w1070:dbl)
                        n1008 = Add(x=w1051, y=w1052) -> (x+y=w1050:dbl)
                        n1009 = local write "Flow Rate"(w1070) -> ()
                        n1010 = stacked-sequence {
                          frame #0 {
                            n1011 = local read "Sum Time"() -> (w1073:dbl)
                            n1012 = local read "Data Sampling Rate (s)"() -> (w1072:dbl)
                            n1013 = Add(x=w1073, y=w1072) -> (x+y=w1071:dbl)
                            n1014 = local write "25%RateTime"(w1071) -> ()
                            n1015 = local write "Sum Time"(w1071) -> ()
                          }
                          frame #1 {
                            n1016 = local read "Sum Time"() -> (w1077:dbl)
                            n1017 = Quotient & Remainder(x=w1077, y=60) -> (x-y*floor(x/y)=w1074:dbl, floor(x/y)=w1075:dbl)
                            n1018 = local write "Minutes"(w1075) -> ()
                            n1019 = local write "Seconds"(w1074) -> ()
                          }
                        }
                        n1020 = local write "Cubic Ft. Flowed"(w1050) -> ()
                      }
                    }
                  }
                  frame 5 {
                    n1021 = stacked-sequence {
                      frame #0 {
                        n1022 = local write "Meter SLPM"(10) -> ()
                        n1023 = local write "Gas Type"("LP") -> ()
                        n1024 = local write "Signal 2"(TRUE) -> ()
                      }
                      frame #1 {
                        n1025 = local read "Gas Type"() -> (w1112:string)
                        n1026 = case shown="\"NG\", Default" w1112 {
                          tunnel: [w1134 w1143] -> w1111
                          tunnel: [TRUE FALSE] -> w1110
                          tunnel: [FALSE TRUE] -> w1109
                          tunnel: [1.0 0.995] -> w1108
                          tunnel: [w1128 w1138] -> w1107
                          frame "LP" {
                            n1027 = local read "Meter SLPM"() -> (w1136:dbl)
                            n1028 = Divide(x=w1136, y=0.5) -> (x/y=w1129:dbl)
                            n1029 = Multiply(x=0.211888, y=w1129) -> (x*y=w1134:dbl)
                            n1030 = local read "HeatingValueLP"() -> (w1128:dbl)
                            n1031 = Multiply(x=w1129, y=2600) -> ()  [unwired: 1 out]
                          }
                          frame "NG", Default {
                            n1032 = local read "Meter SLPM"() -> (w1145:dbl)
                            n1033 = Divide(x=w1145, y=1.0) -> (x/y=w1139:dbl)
                            n1034 = Multiply(x=0.423776, y=w1139) -> (x*y=w1143:dbl)
                            n1035 = local read "HeatingValueNG"() -> (w1138:dbl)
                          }
                        }
                        n1036 = local read "Reference5"() -> (w1115:dbl)
                        n1037 = local read "Output 5"() -> (w1116:dbl)
                        n1038 = Divide(x=w1116, y=w1115) -> (x/y=w1113:dbl)
                        n1039 = Compound Arithmetic op=MULTIPLY(w1113, 5.0, w1111) -> (w1106:dbl)
                        n1040 = local write "CF HR"(w1106) -> ()
                        n1041 = Divide(x=w1106, y=3600) -> (x/y=w1104:dbl)
                        n1042 = local read "CF HR"() -> (w1117:dbl)
                        n1043 = local read "HV"() -> (w1118:dbl)
                        n1044 = Multiply(x=0.025, y=w1104) -> (x*y=w1101:dbl)
                        n1045 = local write "HV"(w1107) -> ()
                        n1046 = Multiply(x=w1117, y=w1118) -> (x*y=w1119:dbl)
                        n1047 = local read "Cubic Ft. Flowed"() -> (w1102:dbl)
                        n1048 = property on="HeatingValueNG" class="DigNum (strict)"("Visible"=w1109) -> ()  [unwired: 2 in, 2 out]
                        n1049 = property on="HeatingValueLP" class="DigNum (strict)"("Visible"=w1110) -> ()  [unwired: 2 in, 2 out]
                        n1050 = Multiply(x=w1119, y=w1108) -> (x*y=w1120:dbl)
                        n1051 = Add(x=w1101, y=w1102) -> (x+y=w1100:dbl)
                        n1052 = local write "Flow Rate"(w1120) -> ()
                        n1053 = stacked-sequence {
                          frame #0 {
                            n1054 = local read "Sum Time"() -> (w1123:dbl)
                            n1055 = local read "Data Sampling Rate (s)"() -> (w1122:dbl)
                            n1056 = Add(x=w1123, y=w1122) -> (x+y=w1121:dbl)
                            n1057 = local write "25%RateTime"(w1121) -> ()
                            n1058 = local write "Sum Time"(w1121) -> ()
                          }
                          frame #1 {
                            n1059 = local read "Sum Time"() -> (w1127:dbl)
                            n1060 = Quotient & Remainder(x=w1127, y=60) -> (x-y*floor(x/y)=w1124:dbl, floor(x/y)=w1125:dbl)
                            n1061 = local write "Minutes"(w1125) -> ()
                            n1062 = local write "Seconds"(w1124) -> ()
                          }
                        }
                        n1063 = local write "Cubic Ft. Flowed"(w1100) -> ()
                      }
                    }
                  }
                  frame 6 {
                    n1064 = stacked-sequence {
                      frame #0 {
                        n1065 = local write "Meter SLPM"(20) -> ()
                        n1066 = local write "Gas Type"("LP") -> ()
                        n1067 = local write "Signal 2"(TRUE) -> ()
                      }
                      frame #1 {
                        n1068 = local read "Gas Type"() -> (w1162:string)
                        n1069 = case shown="\"NG\", Default" w1162 {
                          tunnel: [w1184 w1193] -> w1161
                          tunnel: [TRUE FALSE] -> w1160
                          tunnel: [FALSE TRUE] -> w1159
                          tunnel: [1.0 0.995] -> w1158
                          tunnel: [w1178 w1188] -> w1157
                          frame "LP" {
                            n1070 = local read "Meter SLPM"() -> (w1186:dbl)
                            n1071 = Divide(x=w1186, y=0.5) -> (x/y=w1179:dbl)
                            n1072 = Multiply(x=0.211888, y=w1179) -> (x*y=w1184:dbl)
                            n1073 = local read "HeatingValueLP"() -> (w1178:dbl)
                            n1074 = Multiply(x=w1179, y=2600) -> ()  [unwired: 1 out]
                          }
                          frame "NG", Default {
                            n1075 = local read "Meter SLPM"() -> (w1195:dbl)
                            n1076 = Divide(x=w1195, y=1.0) -> (x/y=w1189:dbl)
                            n1077 = Multiply(x=0.423776, y=w1189) -> (x*y=w1193:dbl)
                            n1078 = local read "HeatingValueNG"() -> (w1188:dbl)
                          }
                        }
                        n1079 = local read "Reference6"() -> (w1165:dbl)
                        n1080 = local read "Output 6"() -> (w1166:dbl)
                        n1081 = Divide(x=w1166, y=w1165) -> (x/y=w1163:dbl)
                        n1082 = Compound Arithmetic op=MULTIPLY(w1163, 5.0, w1161) -> (w1156:dbl)
                        n1083 = local write "CF HR"(w1156) -> ()
                        n1084 = Divide(x=w1156, y=3600) -> (x/y=w1154:dbl)
                        n1085 = local read "CF HR"() -> (w1167:dbl)
                        n1086 = local read "HV"() -> (w1168:dbl)
                        n1087 = Multiply(x=0.025, y=w1154) -> (x*y=w1151:dbl)
                        n1088 = local write "HV"(w1157) -> ()
                        n1089 = Multiply(x=w1167, y=w1168) -> (x*y=w1169:dbl)
                        n1090 = local read "Cubic Ft. Flowed"() -> (w1152:dbl)
                        n1091 = property on="HeatingValueNG" class="DigNum (strict)"("Visible"=w1159) -> ()  [unwired: 2 in, 2 out]
                        n1092 = property on="HeatingValueLP" class="DigNum (strict)"("Visible"=w1160) -> ()  [unwired: 2 in, 2 out]
                        n1093 = Multiply(x=w1169, y=w1158) -> (x*y=w1170:dbl)
                        n1094 = Add(x=w1151, y=w1152) -> (x+y=w1150:dbl)
                        n1095 = stacked-sequence {
                          frame #0 {
                            n1096 = local read "Data Sampling Rate (s)"() -> (w1172:dbl)
                            n1097 = local read "Sum Time"() -> (w1173:dbl)
                            n1098 = Add(x=w1173, y=w1172) -> (x+y=w1171:dbl)
                            n1099 = local write "25%RateTime"(w1171) -> ()
                            n1100 = local write "Sum Time"(w1171) -> ()
                          }
                          frame #1 {
                            n1101 = local read "Sum Time"() -> (w1177:dbl)
                            n1102 = Quotient & Remainder(x=w1177, y=60) -> (x-y*floor(x/y)=w1174:dbl, floor(x/y)=w1175:dbl)
                            n1103 = local write "Minutes"(w1175) -> ()
                            n1104 = local write "Seconds"(w1174) -> ()
                          }
                        }
                        n1105 = local write "Flow Rate"(w1170) -> ()
                        n1106 = local write "Cubic Ft. Flowed"(w1150) -> ()
                      }
                    }
                  }
                }
              }
            }
            n1107 = call-poly <vilib>:"DAQmx Read.vi"("task/channels in"=w893) -> ("data"=w892:dbl[])  [unwired: 12 in, 2 out]
            n1108 = Index Array(array=w892, index=8) -> (element=w876:dbl)
            n1109 = Index Array(array=w892, index=5) -> (element=w873:dbl)
            n1110 = Index Array(array=w892, index=6) -> (element=w874:dbl)
            n1111 = Index Array(array=w892, index=7) -> (element=w875:dbl)
            n1112 = Index Array(array=w892, index=4) -> (element=w872:dbl)
            n1113 = Index Array(array=w892, index=0) -> (element=w868:dbl)
            n1114 = Index Array(array=w892, index=1) -> (element=w869:dbl)
            n1115 = Index Array(array=w892, index=3) -> (element=w871:dbl)
            n1116 = Index Array(array=w892, index=2) -> (element=w870:dbl)
            n1117 = local write "Output 3"(w876) -> ()
            n1118 = local write "Output 2"(w875) -> ()
            n1119 = local write "Output 1"(w874) -> ()
            n1120 = local write "Reference1"(w868) -> ()
            n1121 = local write "Reference6"(w873) -> ()
            n1122 = local write "Reference2"(w869) -> ()
            n1123 = local write "Reference4"(w871) -> ()
            n1124 = local write "Reference3"(w870) -> ()
            n1125 = local write "Reference5"(w872) -> ()
            n1126 = Index Array(array=w892, index=9) -> (element=w877:dbl)
            n1127 = Index Array(array=w892, index=11) -> (element=w879:dbl)
            n1128 = Index Array(array=w892, index=10) -> (element=w878:dbl)
            n1129 = local write "Output 6"(w879) -> ()
            n1130 = local write "Output 5"(w878) -> ()
            n1131 = local write "Output 4"(w877) -> ()
          }
        }
      }
    }
  }
